vi "Text control 2 v5.0_pump-specific.vi"() -> ()   [LabVIEW 2016]
panel:
  in  "Tab Control":enum32{"Main", "Other parameters"}(tab)
  out "Line running":i32
  out "Total lines":i32
  out "Path":path=path "C:/users/rlp38/09Apr2009LTtesting/test2.txt"
  out "I vs Vg":cluster{"Y data in":dbl[], "X data in":dbl[]}[](graph)
  out "Is":dbl format="%.2e"
  out "Id":dbl format="%.2e"
  out "Ig":dbl format="%.2e"
  out "Id max vs time":cluster{"Y data in":dbl[], "X data in":dbl[]}[](graph)
  out "Id min vs time":cluster{"Y data in":dbl[], "X data in":dbl[]}[](graph)
  out "I vs Vd":cluster{"Y data in":dbl[], "X data in":dbl[]}[](graph)
  in  "Program":string="#-------------------------------------------------------\n# Liquid cycling script\n# Version 0.1\n# Author: Dimitrios Simatos\n# Last updated: 2017-10-12\n#-------------------------------------------------------\n# Things to do before running the script:\n# Set time units to minutes.\n# Set filenames.\n# Replace the tubing, if necessary.\n#-------------------------------------------------------\n# Port connections\n# Port 1: Waste\n# Port 2: Device\n# Port 3: Ultrapure water\n# Port 4: Nothing\n# Port 5: Nothing\n# Port 6: Nothing\n#-------------------------------------------------------\n# Execution time: 4 x 30 = 120 minutes = 2 hours\n# This script is designed to perform a cycling experiment between two liquids.\n# There are 4 pumping cycles, each one followed by 30 minutes of measurements.\n# All cycles pump ultrapure water (port 3).\n# Flow V = 20 pulses/second (400 ul/min)\n#-------------------------------------------------------\n# Cycle 1\npump /1ZR #initialize pump\npump /1Q #query pump\ntransfer d 1 -1 -0.1 -1 -1 0\npump /1? #report absolute plunger position\npump /1?6 #report valve position\nwait-min 1 #wait 1 minute\ntransfer d 1 -1 -0.1 -1 -1 0\npump /1N0R #set step resolution: 0.01 mm\npump /1Q #query pump\npump /1? #report absolute plunger position (the plunger should be at 0)\npump /1?6 #report valve position\nwait 1000 #wait 1 second\npump /1V300R #choose speed: 300 steps/s\npump /1Q #query pump\nwait 1000 #wait 1 second\npump /1O3R #go to port 3, counterclockwise rotation\npump /1Q #query pump\nwait 1000 #wait 1 second\npump /1A2400R #go to absolute position 2400\nwait 20000 #wait 20 seconds\npump /1V20R #set speed to 20 steps/s\npump /1Q #query pump\nwait 10000 # wait 10 seconds\ntransfer d 1 -1 -0.1 -1 -1 0\npump /1? #report absolute plunger position (the plunger should have finished moving)\npump /1?6 #report valve position\npump /1O2R #switch to port 2, counterclockwise rotation\npump /1Q #query pump\nwait 200 #wait 200 milliseconds\npump /1A0R #go to absolute position 0 (= empty syringe)\npump /1Q #query pump\npump /1? #report absolute plunger position (the plunger should be moving to 0)\npump /1?6 #report valve position\ntransfer d 1 -1 -0.1 -1 -1 0\nwait-min 1\npump /1Q #query pump\npump /1? #report absolute plunger position (the plunger should be moving to 0)\npump /1?6 #report valve position\ntransfer d 1 -1 -0.1 -1 -1 0\nwait-min 1\npump /1Q #query pump\npump /1? #report absolute plunger position\npump /1?6 #report valve position\ntransfer d 1 -1 -0.1 -1 -1 0\nwait-min 1\npump /1Q #query pump\npump /1? #report absolute plunger position\npump /1?6 #report valve position\ntransfer d 1 -1 -0.1 -1 -1 0\nwait-min 1\npump /1Q #query pump\npump /1? #report absolute plunger position\npump /1?6 #report valve position\ntransfer d 1 -1 -0.1 -1 -1 0\nwait-min 1\npump /1Q #query pump\npump /1? #report absolute plunger position\npump /1?6 #report valve position\ntransfer d 1 -1 -0.1 -1 -1 0\nwait-min 1\npump /1Q #query pump\npump /1? #report absolute plunger position\npump /1?6 #report valve position\ntransfer d 1 -1 -0.1 -1 -1 0\nwait-min 1\npump /1Q #query pump\npump /1? #report absolute plunger position\npump /1?6 #report valve position\ntransfer d 1 -1 -0.1 -1 -1 0\nwait-min 1\npump /1Q #query pump\npump /1? #report absolute plunger position\npump /1?6 #report valve position\ntransfer d 1 -1 -0.1 -1 -1 0\nwait-min 1\npump /1Q #query pump\npump /1? #report absolute plunger position\npump /1?6 #report valve position\ntransfer d 1 -1 -0.1 -1 -1 0\nwait-min 1\npump /1Q #query pump\npump /1? #report absolute plunger position\npump /1?6 #report valve position\ntransfer d 1 -1 -0.1 -1 -1 0\nwait-min 1\npump /1Q #query pump\npump /1? #report absolute plunger position\npump /1?6 #report valve position\ntransfer d 1 -1 -0.1 -1 -1 0\nwait-min 1\npump /1Q #query pump\npump /1? #report absolute plunger position\npump /1?6 #report valve position\ntransfer d 1 -1 -0.1 -1 -1 0\nwait-min 1\npump /1Q #query pump\npump /1? #report absolute plunger position\npump /1?6 #report valve position\ntransfer d 1 -1 -0.1 -1 -1 0\nwait-min 1\npump /1Q #query pump\npump /1? #report absolute plunger position\npump /1?6 #report valve position\ntransfer d 1 -1 -0.1 -1 -1 0\nwait-min 1\npump /1Q #query pump\npump /1? #report absolute plunger position\npump /1?6 #report valve position\ntransfer d 1 -1 -0.1 -1 -1 0\nwait-min 1\npump /1Q #query pump\npump /1? #report absolute plunger position\npump /1?6 #report valve position\ntransfer d 1 -1 -0.1 -1 -1 0\nwait-min 1\npump /1Q #query pump\npump /1? #report absolute plunger position\npump /1?6 #report valve position\ntransfer d 1 -1 -0.1 -1 -1 0\nwait-min 1\npump /1Q #query pump\npump /1? #report absolute plunger position\npump /1?6 #report valve position\ntransfer d 1 -1 -0.1 -1 -1 0\nwait-min 1\npump /1Q #query pump\npump /1? #report absolute plunger position\npump /1?6 #report valve position\ntransfer d 1 -1 -0.1 -1 -1 0\nwait-min 1\npump /1Q #query pump\npump /1? #report absolute plunger position\npump /1?6 #report valve position\ntransfer d 1 -1 -0.1 -1 -1 0\nwait-min 1\npump /1Q #query pump\npump /1? #report absolute plunger position\npump /1?6 #report valve position\ntransfer d 1 -1 -0.1 -1 -1 0\nwait-min 1\npump /1Q #query pump\npump /1? #report absolute plunger position\npump /1?6 #report valve position\ntransfer d 1 -1 -0.1 -1 -1 0\nwait-min 1\npump /1Q #query pump\npump /1? #report absolute plunger position\npump /1?6 #report valve position\ntransfer d 1 -1 -0.1 -1 -1 0\nwait-min 1\npump /1Q #query pump\npump /1? #report absolute plunger position\npump /1?6 #report valve position\ntransfer d 1 -1 -0.1 -1 -1 0\nwait-min 1\n#-------------------------------------------------------\n# Cycle 2\npump /1ZR #initialize pump\npump /1Q #query pump\ntransfer d 1 -1 -0.1 -1 -1 0\npump /1? #report absolute plunger position\npump /1?6 #report valve position\nwait-min 1 #wait 1 minute\ntransfer d 1 -1 -0.1 -1 -1 0\npump /1N0R #set step resolution: 0.01 mm\npump /1Q #query pump\npump /1? #report absolute plunger position (the plunger should be at 0)\npump /1?6 #report valve position\nwait 1000 #wait 1 second\npump /1V300R #choose speed: 300 steps/s\npump /1Q #query pump\nwait 1000 #wait 1 second\npump /1O3R #go to port 3, counterclockwise rotation\npump /1Q #query pump\nwait 1000 #wait 1 second\npump /1A2400R #go to absolute position 2400\nwait 20000 #wait 20 seconds\ntransfer d 1 -1 -0.1 -1 -1 0\npump /1V20R #set speed to 20 steps/s\npump /1Q #query pump\nwait 10000 # wait 10 seconds\npump /1? #report absolute plunger position (the plunger should have finished moving)\npump /1?6 #report valve position\npump /1O2R #switch to port 2, counterclockwise rotation\npump /1Q #query pump\nwait 200 #wait 200 milliseconds\npump /1A0R #go to absolute position 0 (= empty syringe)\npump /1Q #query pump\npump /1? #report absolute plunger position (the plunger should be moving to 0)\npump /1?6 #report valve position\ntransfer d 1 -1 -0.1 -1 -1 0\nwait-min 1\npump /1Q #query pump\npump /1? #report absolute plunger position (the plunger should be moving to 0)\npump /1?6 #report valve position\ntransfer d 1 -1 -0.1 -1 -1 0\nwait-min 1\npump /1Q #query pump\npump /1? #report absolute plunger position\npump /1?6 #report valve position\ntransfer d 1 -1 -0.1 -1 -1 0\nwait-min 1\npump /1Q #query pump\npump /1? #report absolute plunger position\npump /1?6 #report valve position\ntransfer d 1 -1 -0.1 -1 -1 0\nwait-min 1\npump /1Q #query pump\npump /1? #report absolute plunger position\npump /1?6 #report valve position\ntransfer d 1 -1 -0.1 -1 -1 0\nwait-min 1\npump /1Q #query pump\npump /1? #report absolute plunger position\npump /1?6 #report valve position\ntransfer d 1 -1 -0.1 -1 -1 0\nwait-min 1\npump /1Q #query pump\npump /1? #report absolute plunger position\npump /1?6 #report valve position\ntransfer d 1 -1 -0.1 -1 -1 0\nwait-min 1\npump /1Q #query pump\npump /1? #report absolute plunger position\npump /1?6 #report valve position\ntransfer d 1 -1 -0.1 -1 -1 0\nwait-min 1\npump /1Q #query pump\npump /1? #report absolute plunger position\npump /1?6 #report valve position\ntransfer d 1 -1 -0.1 -1 -1 0\nwait-min 1\npump /1Q #query pump\npump /1? #report absolute plunger position\npump /1?6 #report valve position\ntransfer d 1 -1 -0.1 -1 -1 0\nwait-min 1\npump /1Q #query pump\npump /1? #report absolute plunger position\npump /1?6 #report valve position\ntransfer d 1 -1 -0.1 -1 -1 0\nwait-min 1\npump /1Q #query pump\npump /1? #report absolute plunger position\npump /1?6 #report valve position\ntransfer d 1 -1 -0.1 -1 -1 0\nwait-min 1\npump /1Q #query pump\npump /1? #report absolute plunger position\npump /1?6 #report valve position\ntransfer d 1 -1 -0.1 -1 -1 0\nwait-min 1\npump /1Q #query pump\npump /1? #report absolute plunger position\npump /1?6 #report valve position\ntransfer d 1 -1 -0.1 -1 -1 0\nwait-min 1\npump /1Q #query pump\npump /1? #report absolute plunger position\npump /1?6 #report valve position\ntransfer d 1 -1 -0.1 -1 -1 0\nwait-min 1\npump /1Q #query pump\npump /1? #report absolute plunger position\npump /1?6 #report valve position\ntransfer d 1 -1 -0.1 -1 -1 0\nwait-min 1\npump /1Q #query pump\npump /1? #report absolute plunger position\npump /1?6 #report valve position\ntransfer d 1 -1 -0.1 -1 -1 0\nwait-min 1\npump /1Q #query pump\npump /1? #report absolute plunger position\npump /1?6 #report valve position\ntransfer d 1 -1 -0.1 -1 -1 0\nwait-min 1\npump /1Q #query pump\npump /1? #report absolute plunger position\npump /1?6 #report valve position\ntransfer d 1 -1 -0.1 -1 -1 0\nwait-min 1\npump /1Q #query pump\npump /1? #report absolute plunger position\npump /1?6 #report valve position\ntransfer d 1 -1 -0.1 -1 -1 0\nwait-min 1\npump /1Q #query pump\npump /1? #report absolute plunger position\npump /1?6 #report valve position\ntransfer d 1 -1 -0.1 -1 -1 0\nwait-min 1\npump /1Q #query pump\npump /1? #report absolute plunger position\npump /1?6 #report valve position\ntransfer d 1 -1 -0.1 -1 -1 0\nwait-min 1\npump /1Q #query pump\npump /1? #report absolute plunger position\npump /1?6 #report valve position\ntransfer d 1 -1 -0.1 -1 -1 0\nwait-min 1\npump /1Q #query pump\npump /1? #report absolute plunger position\npump /1?6 #report valve position\ntransfer d 1 -1 -0.1 -1 -1 0\nwait-min 1\npump /1Q #query pump\npump /1? #report absolute plunger position\npump /1?6 #report valve position\ntransfer d 1 -1 -0.1 -1 -1 0\nwait-min 1\n#-------------------------------------------------------\n# Cycle 3\npump /1ZR #initialize pump\npump /1Q #query pump\ntransfer d 1 -1 -0.1 -1 -1 0\npump /1? #report absolute plunger position\npump /1?6 #report valve position\nwait-min 1 #wait 1 minute\ntransfer d 1 -1 -0.1 -1 -1 0\npump /1N0R #set step resolution: 0.01 mm\npump /1Q #query pump\npump /1? #report absolute plunger position (the plunger should be at 0)\npump /1?6 #report valve position\nwait 1000 #wait 1 second\npump /1V300R #choose speed: 300 steps/s\npump /1Q #query pump\nwait 1000 #wait 1 second\npump /1O3R #go to port 3, counterclockwise rotation\npump /1Q #query pump\nwait 1000 #wait 1 second\npump /1A2400R #go to absolute position 2400\nwait 20000 #wait 20 seconds\ntransfer d 1 -1 -0.1 -1 -1 0\npump /1V20R #set speed to 20 steps/s\npump /1Q #query pump\nwait 10000 # wait 10 seconds\npump /1? #report absolute plunger position (the plunger should have finished moving)\npump /1?6 #report valve position\npump /1O2R #switch to port 2, counterclockwise rotation\npump /1Q #query pump\nwait 200 #wait 200 milliseconds\npump /1A0R #go to absolute position 0 (= empty syringe)\npump /1Q #query pump\npump /1? #report absolute plunger position (the plunger should be moving to 0)\npump /1?6 #report valve position\ntransfer d 1 -1 -0.1 -1 -1 0\nwait-min 1\npump /1Q #query pump\npump /1? #report absolute plunger position (the plunger should be moving to 0)\npump /1?6 #report valve position\ntransfer d 1 -1 -0.1 -1 -1 0\nwait-min 1\npump /1Q #query pump\npump /1? #report absolute plunger position\npump /1?6 #report valve position\ntransfer d 1 -1 -0.1 -1 -1 0\nwait-min 1\npump /1Q #query pump\npump /1? #report absolute plunger position\npump /1?6 #report valve position\ntransfer d 1 -1 -0.1 -1 -1 0\nwait-min 1\npump /1Q #query pump\npump /1? #report absolute plunger position\npump /1?6 #report valve position\ntransfer d 1 -1 -0.1 -1 -1 0\nwait-min 1\npump /1Q #query pump\npump /1? #report absolute plunger position\npump /1?6 #report valve position\ntransfer d 1 -1 -0.1 -1 -1 0\nwait-min 1\npump /1Q #query pump\npump /1? #report absolute plunger position\npump /1?6 #report valve position\ntransfer d 1 -1 -0.1 -1 -1 0\nwait-min 1\npump /1Q #query pump\npump /1? #report absolute plunger position\npump /1?6 #report valve position\ntransfer d 1 -1 -0.1 -1 -1 0\nwait-min 1\npump /1Q #query pump\npump /1? #report absolute plunger position\npump /1?6 #report valve position\ntransfer d 1 -1 -0.1 -1 -1 0\nwait-min 1\npump /1Q #query pump\npump /1? #report absolute plunger position\npump /1?6 #report valve position\ntransfer d 1 -1 -0.1 -1 -1 0\nwait-min 1\npump /1Q #query pump\npump /1? #report absolute plunger position\npump /1?6 #report valve position\ntransfer d 1 -1 -0.1 -1 -1 0\nwait-min 1\npump /1Q #query pump\npump /1? #report absolute plunger position\npump /1?6 #report valve position\ntransfer d 1 -1 -0.1 -1 -1 0\nwait-min 1\npump /1Q #query pump\npump /1? #report absolute plunger position\npump /1?6 #report valve position\ntransfer d 1 -1 -0.1 -1 -1 0\nwait-min 1\npump /1Q #query pump\npump /1? #report absolute plunger position\npump /1?6 #report valve position\ntransfer d 1 -1 -0.1 -1 -1 0\nwait-min 1\npump /1Q #query pump\npump /1? #report absolute plunger position\npump /1?6 #report valve position\ntransfer d 1 -1 -0.1 -1 -1 0\nwait-min 1\npump /1Q #query pump\npump /1? #report absolute plunger position\npump /1?6 #report valve position\ntransfer d 1 -1 -0.1 -1 -1 0\nwait-min 1\npump /1Q #query pump\npump /1? #report absolute plunger position\npump /1?6 #report valve position\ntransfer d 1 -1 -0.1 -1 -1 0\nwait-min 1\npump /1Q #query pump\npump /1? #report absolute plunger position\npump /1?6 #report valve position\ntransfer d 1 -1 -0.1 -1 -1 0\nwait-min 1\npump /1Q #query pump\npump /1? #report absolute plunger position\npump /1?6 #report valve position\ntransfer d 1 -1 -0.1 -1 -1 0\nwait-min 1\npump /1Q #query pump\npump /1? #report absolute plunger position\npump /1?6 #report valve position\ntransfer d 1 -1 -0.1 -1 -1 0\nwait-min 1\npump /1Q #query pump\npump /1? #report absolute plunger position\npump /1?6 #report valve position\ntransfer d 1 -1 -0.1 -1 -1 0\nwait-min 1\npump /1Q #query pump\npump /1? #report absolute plunger position\npump /1?6 #report valve position\ntransfer d 1 -1 -0.1 -1 -1 0\nwait-min 1\npump /1Q #query pump\npump /1? #report absolute plunger position\npump /1?6 #report valve position\ntransfer d 1 -1 -0.1 -1 -1 0\nwait-min 1\npump /1Q #query pump\npump /1? #report absolute plunger position\npump /1?6 #report valve position\ntransfer d 1 -1 -0.1 -1 -1 0\nwait-min 1\npump /1Q #query pump\npump /1? #report absolute plunger position\npump /1?6 #report valve position\ntransfer d 1 -1 -0.1 -1 -1 0\nwait-min 1\n#-------------------------------------------------------\n# Cycle 4\npump /1ZR #initialize pump\npump /1Q #query pump\ntransfer d 1 -1 -0.1 -1 -1 0\npump /1? #report absolute plunger position\npump /1?6 #report valve position\nwait-min 1 #wait 1 minute\ntransfer d 1 -1 -0.1 -1 -1 0\npump /1N0R #set step resolution: 0.01 mm\npump /1Q #query pump\npump /1? #report absolute plunger position (the plunger should be at 0)\npump /1?6 #report valve position\nwait 1000 #wait 1 second\npump /1V300R #choose speed: 300 steps/s\npump /1Q #query pump\nwait 1000 #wait 1 second\npump /1O3R #go to port 3, counterclockwise rotation\npump /1Q #query pump\nwait 1000 #wait 1 second\npump /1A2400R #go to absolute position 2400\nwait 20000 #wait 20 seconds\ntransfer d 1 -1 -0.1 -1 -1 0\npump /1V20R #set speed to 20 steps/s\npump /1Q #query pump\nwait 10000 # wait 10 seconds\npump /1? #report absolute plunger position (the plunger should have finished moving)\npump /1?6 #report valve position\npump /1O2R #switch to port 2, counterclockwise rotation\npump /1Q #query pump\nwait 200 #wait 200 milliseconds\npump /1A0R #go to absolute position 0 (= empty syringe)\npump /1Q #query pump\npump /1? #report absolute plunger position (the plunger should be moving to 0)\npump /1?6 #report valve position\ntransfer d 1 -1 -0.1 -1 -1 0\nwait-min 1\npump /1Q #query pump\npump /1? #report absolute plunger position (the plunger should be moving to 0)\npump /1?6 #report valve position\ntransfer d 1 -1 -0.1 -1 -1 0\nwait-min 1\npump /1Q #query pump\npump /1? #report absolute plunger position\npump /1?6 #report valve position\ntransfer d 1 -1 -0.1 -1 -1 0\nwait-min 1\npump /1Q #query pump\npump /1? #report absolute plunger position\npump /1?6 #report valve position\ntransfer d 1 -1 -0.1 -1 -1 0\nwait-min 1\npump /1Q #query pump\npump /1? #report absolute plunger position\npump /1?6 #report valve position\ntransfer d 1 -1 -0.1 -1 -1 0\nwait-min 1\npump /1Q #query pump\npump /1? #report absolute plunger position\npump /1?6 #report valve position\ntransfer d 1 -1 -0.1 -1 -1 0\nwait-min 1\npump /1Q #query pump\npump /1? #report absolute plunger position\npump /1?6 #report valve position\ntransfer d 1 -1 -0.1 -1 -1 0\nwait-min 1\npump /1Q #query pump\npump /1? #report absolute plunger position\npump /1?6 #report valve position\ntransfer d 1 -1 -0.1 -1 -1 0\nwait-min 1\npump /1Q #query pump\npump /1? #report absolute plunger position\npump /1?6 #report valve position\ntransfer d 1 -1 -0.1 -1 -1 0\nwait-min 1\npump /1Q #query pump\npump /1? #report absolute plunger position\npump /1?6 #report valve position\ntransfer d 1 -1 -0.1 -1 -1 0\nwait-min 1\npump /1Q #query pump\npump /1? #report absolute plunger position\npump /1?6 #report valve position\ntransfer d 1 -1 -0.1 -1 -1 0\nwait-min 1\npump /1Q #query pump\npump /1? #report absolute plunger position\npump /1?6 #report valve position\ntransfer d 1 -1 -0.1 -1 -1 0\nwait-min 1\npump /1Q #query pump\npump /1? #report absolute plunger position\npump /1?6 #report valve position\ntransfer d 1 -1 -0.1 -1 -1 0\nwait-min 1\npump /1Q #query pump\npump /1? #report absolute plunger position\npump /1?6 #report valve position\ntransfer d 1 -1 -0.1 -1 -1 0\nwait-min 1\npump /1Q #query pump\npump /1? #report absolute plunger position\npump /1?6 #report valve position\ntransfer d 1 -1 -0.1 -1 -1 0\nwait-min 1\npump /1Q #query pump\npump /1? #report absolute plunger position\npump /1?6 #report valve position\ntransfer d 1 -1 -0.1 -1 -1 0\nwait-min 1\npump /1Q #query pump\npump /1? #report absolute plunger position\npump /1?6 #report valve position\ntransfer d 1 -1 -0.1 -1 -1 0\nwait-min 1\npump /1Q #query pump\npump /1? #report absolute plunger position\npump /1?6 #report valve position\ntransfer d 1 -1 -0.1 -1 -1 0\nwait-min 1\npump /1Q #query pump\npump /1? #report absolute plunger position\npump /1?6 #report valve position\ntransfer d 1 -1 -0.1 -1 -1 0\nwait-min 1\npump /1Q #query pump\npump /1? #report absolute plunger position\npump /1?6 #report valve position\ntransfer d 1 -1 -0.1 -1 -1 0\nwait-min 1\npump /1Q #query pump\npump /1? #report absolute plunger position\npump /1?6 #report valve position\ntransfer d 1 -1 -0.1 -1 -1 0\nwait-min 1\npump /1Q #query pump\npump /1? #report absolute plunger position\npump /1?6 #report valve position\ntransfer d 1 -1 -0.1 -1 -1 0\nwait-min 1\npump /1Q #query pump\npump /1? #report absolute plunger position\npump /1?6 #report valve position\ntransfer d 1 -1 -0.1 -1 -1 0\nwait-min 1\npump /1Q #query pump\npump /1? #report absolute plunger position\npump /1?6 #report valve position\ntransfer d 1 -1 -0.1 -1 -1 0\nwait-min 1\npump /1Q #query pump\npump /1? #report absolute plunger position\npump /1?6 #report valve position\ntransfer d 1 -1 -0.1 -1 -1 0\nwait-min 1\n#-------------------------------------------------------"
  out "Command running:":string="#output s 0 0 0 -0.008 0.008 0.002"
  out "Serial port data":string
  out "Elapsed Time":dbl caption="Elapsed Time (s)"
  in  "Units":u16(ring)=1 items=["Seconds", "Minutes", "Hours"]
  in  "Time Offset":dbl caption="Set Start Time (s)"
  in  "Reset":bool
  in  "Auto Reset":bool
  in  "integration time":u32(slide) max=2 step=1 scale=0.0..2.0
  in  "Interrupt run":bool
  out "Absolute plunger position vs time":cluster{"Y data in":dbl[], "X data in":dbl[]}[](graph)
  out "Valve position vs time":cluster{"Y data in":dbl[], "X data in":dbl[]}[](graph)
  in  "Halt pump":bool
  in  "Hard stop pump":bool
  in  "Gate Range\nmode":u16(ring) items=["Auto", "Limited", "Fixed"]
  in  "Gate Range":u8(slide)=6 max=11 scale=0.0..11.0
  in  "Source/Drain\nRange mode":u16(ring) items=["Auto", "Limited", "Fixed"]
  in  "Source/Drain Range":u8(slide)=6 max=11 scale=0.0..11.0
  in  "Panel Controls":T1={"Emergency Stop"=refnum, "TransGraph Max"=1e-05, "Text/Graph (text=false)"=TRUE} {"TransGraph Max" format="%.2e"}
  in  "Panel Controls 2":T2={"Emergency Stop"=refnum, "TransGraph Max"=1e-05, "Text/Graph (text=false)"=TRUE, "TransGraph Min"=1e-11} {"TransGraph Min" format="%.2e"; "TransGraph Max" format="%.2e"}
  in  "SMU4":cluster{"on/off":bool, "Voltage":dbl} {"Voltage" min=-100.0 max=100.0 format="%.2f"}
  in  "Full Reset":bool
  in  "Standby":T3
  out "error out":errorcluster
  in  "Delay before read (ms)":u32=1000
  in  "byte count":u32=64
  in  "Serial End Mode for Reads":u16(ring)=2 items=["None", "LastBit", "TermChar"]
  in  "Timeout (ms)":u32=10000
  in  "Enable Termination\nChar (T)":bool=TRUE
  in  "Termination char\n(0xA = '\\n' = LF)\n(0xD = '\\r' = CR)":u8=13 format="%.0x"
  in  "flow control":u16(ring) items=["None"=0, "XON/XOFF"=1, "RTS/CTS"=2, "DTR/DSR"=4]
  in  "stop bits":u16(ring)=10 items=["1.0"=10, "1.5"=15, "2.0"=20]
  in  "parity":u16(ring) items=["None", "Odd", "Even", "Mark", "Space"]
  in  "data bits":u16=8 min=5 max=8 step=1
  in  "VISA resource name":refnum<visa-resource-name>="COM6"
  in  "baud rate":u32=9600
  in  "Drain: Compliance":dbl=0.001 format="%.8f"
  in  "Gate: Compliance":dbl=0.001 format="%.8f"
  in  "hold time /s":dbl format="%.2f"
  in  "delay time /s":dbl format="%.2f"
  in  "Integration time (short)":dbl=0.0019 min=8e-05 max=0.0019 step=8e-05 format="%^.0e"
  in  "Integration time (long)":dbl=0.32 min=0.04 max=2.0 step=0.02 format="%.2f"
  in  "Step delay /s":dbl format="%.2f"
  in  "Prefix (transfer)":string="_step_1_ultrapure_H2O_"
  in  "Suffix (transfer)":string="_T.txt"
  in  "Prefix (Idmax-Idmin)":string="_step_1_ultrapure_H2O_Idmax_Idmin_vs_time_Vg=-1.0V_Vd=-1.0V"
  in  "Suffix (Idmax-Idmin)":string=".txt"
  in  "Prefix (output)":string="_step_1_ultrapure_H2O_"
  in  "Suffix (output)":string="_O.txt"
  in  "Prefix (script)":string="_step_1_ultrapure_H2O_script"
  in  "Prefix (serial port log)":string="_step_1_ultrapure_H2O_serial port output"
  in  "Prefix (plunger)":string="_step_1_ultrapure_H2O_plunger_vs_time"
  in  "Suffix (plunger)":string=".txt"
  in  "Prefix (valve)":string="_step_1_ultrapure_H2O_valve_vs_time"
  in  "Suffix (valve)":string=".txt"
  in  "Gate":T4={"Gate Start"=0.0, "Gate Stop"=2.0, "Gate Step (linear only)"=1.0, "Gate Compliance"=0.0001, "Gate PComp"=0.0, "Range mode"=0, "Range"=6} {"Range" max=11 scale=0.0..11.0; "Range mode" items=["Auto", "Limited", "Fixed"]; "Gate PComp" format="%^.2e"; "Gate Compliance" format="%^.2e"; "Gate Step (linear only)" format="%^.4e"; "Gate Stop" format="%^.4e"; "Gate Start" format="%^.4e"}
  in  "Drain 2":T5={"Drain Start"=0.0, "Drain Stop"=2.0, "Drain Compliance"=0.0001, "Drain Step"=1.0, "Drain PComp"=0.0, "Range mode"=0, "Range"=6} {"Range" max=11 scale=0.0..11.0; "Range mode" items=["Auto", "Limited", "Fixed"]; "Drain PComp" format="%^.2e"; "Drain Step" format="%^.4e"; "Drain Compliance" format="%^.2e"; "Drain Stop" format="%^.4e"; "Drain Start" format="%^.4e"}
  in  "Timings 2":T6={"integration time"=0, "Short/Long integration time"=0.00064, "hold time (sec)"=0.0, "delay time (sec)"=0.0, "Step Time (0 disables)"=0.0, "sweep method"=0, "Pulse period"=0.005, "Base voltage"=0.0, "Pulse width"=0.0005} {"Pulse width" min=0.0005 max=0.1 step=0.0001 format="%.4f"; "Base voltage" format="%^.4e"; "Pulse period" min=0.005 max=1.0 step=0.0001 format="%.4f"; "sweep method" items=["Continuous", "Pulsed"]; "Step Time (0 disables)" format="%.2f"; "delay time (sec)" format="%.4f"; "hold time (sec)" format="%.4f"; "Short/Long integration time" format="%^.0e"; "integration time" scale=0.0..2.0}
  # "Syntax:\nitime [s|m|l]\ngaterangemode [a|l|f]\ndrainrangemode [a|l|f]\npulsed [on|off] PulsePeriod(sec) PulseBaseVoltage PulseONWidth(sec)\nstandby [on l off]\nwait NumMilliseconds\nwait-min NumMinutes\n# texthere = comment\ntransfer [s|d] VgStart VgStop VgStep VdStart VdStop VdStep\noutput [s|d] VgStart VgStop VgStep VdStart VdStop VdStep\nsample Vg Vd NumSamples Time(s) SampleInterval(s)\nsamplei Idg NumSamples Time(s) SampleInterval(s) VDGcompliance\n100 samples is approximately 13 seconds with medium integration\n# if in doubt use SampleInterval(s) = 0.004\nstressV VG VD IGcompliance IDcompliance Duration(sec)\nstressI IDG VDGcompliance Duration(sec)\nvsu2pulse Bias Duration(s)\npulsedstressV [s|d] VEstop VgON VgOFF Period(s) PulseONwidth(s) Vd\nsample-fpp Vg Vd NumSamples Time\nresample-fpp Vg Vd\ntransfer-fpp [s|d] VgStart VgStop VgStep VdStart VdStop VdStep\noutput-fpp [s|d] VgStart VgStop VgStep VdStart VdStop VdStep\nserial SerialPortCommand\npump SerialPortCommand for the OEM pump\n\nSPM OEM Pump Syntax (<x>: pump number, use 1 if only one pump):\nif the command syntax contains [R], then append the letter R to the command\n/<x>Q: query (a query command should follow each command)\n/<x>Z[R] or /<x>Y[R]: initialize pump\n/<x>N<n>[R] (<n>=0,1): <0> (<1>) microstep 0.01 mm (0.00125 mm) resolution\n/<x>I<n> (<n>=0-6): turn to port number n (clockwise)\n/<x>O<n> (<n>=0-6): turn to port number n (counterclockwise)\n/<x>X: Re-execute last command string\n/<x>G<n>[R] (<n>=0-60000): repeat command sequence (default: 0, 0=loop forever)\n/<x>g: Mark the start of a repeat sequence (max = 10)\n/<x>M<n>[R] (<n>=0-86400000): delay command execution by n milliseconds\n/<x>H: Halt; Pause the sequence after finishing the current move\n/<x>T: Hardstop; Interrupt the current move and suppress it from the sequence\n/<x>A<n>[R] (<n>=0-3000 with N=0, 0-24000 with N=1): absolute position\n/<x>P<n>[R] (<n>=0-3000 with N=0, 0-24000 with N=1): relative pickup\n/<x>D<n>[R] (<n>=0-3000 with N=0, 0-24000 with N=1): relative dispense\n/<x>V<n>[R] (<n>=5-1600 default: 150): set peak speed (pulses/sec)\n/<x>S<n>[R] (<n>=10-40 default: 22): set speed (NOT in pulses/sec, look in manual)\nNOTE: When controlled with absolute position, one does not need to pay special attention to the syringe that is mounted on the pump.\nWithdraw from lower stage (ports 3, 5), dispense from higher stage (ports 2, 4, 6).\nConnect Port 1 to waste."
  # "Time"
  # "1\n2\n3\n4\n5\n6\n7\n8\n9\n10\n11\n12\n13\n14\n15\n16\n17\n18\n19\n20"
  # "Serial port settings"
  # "Filename settings"
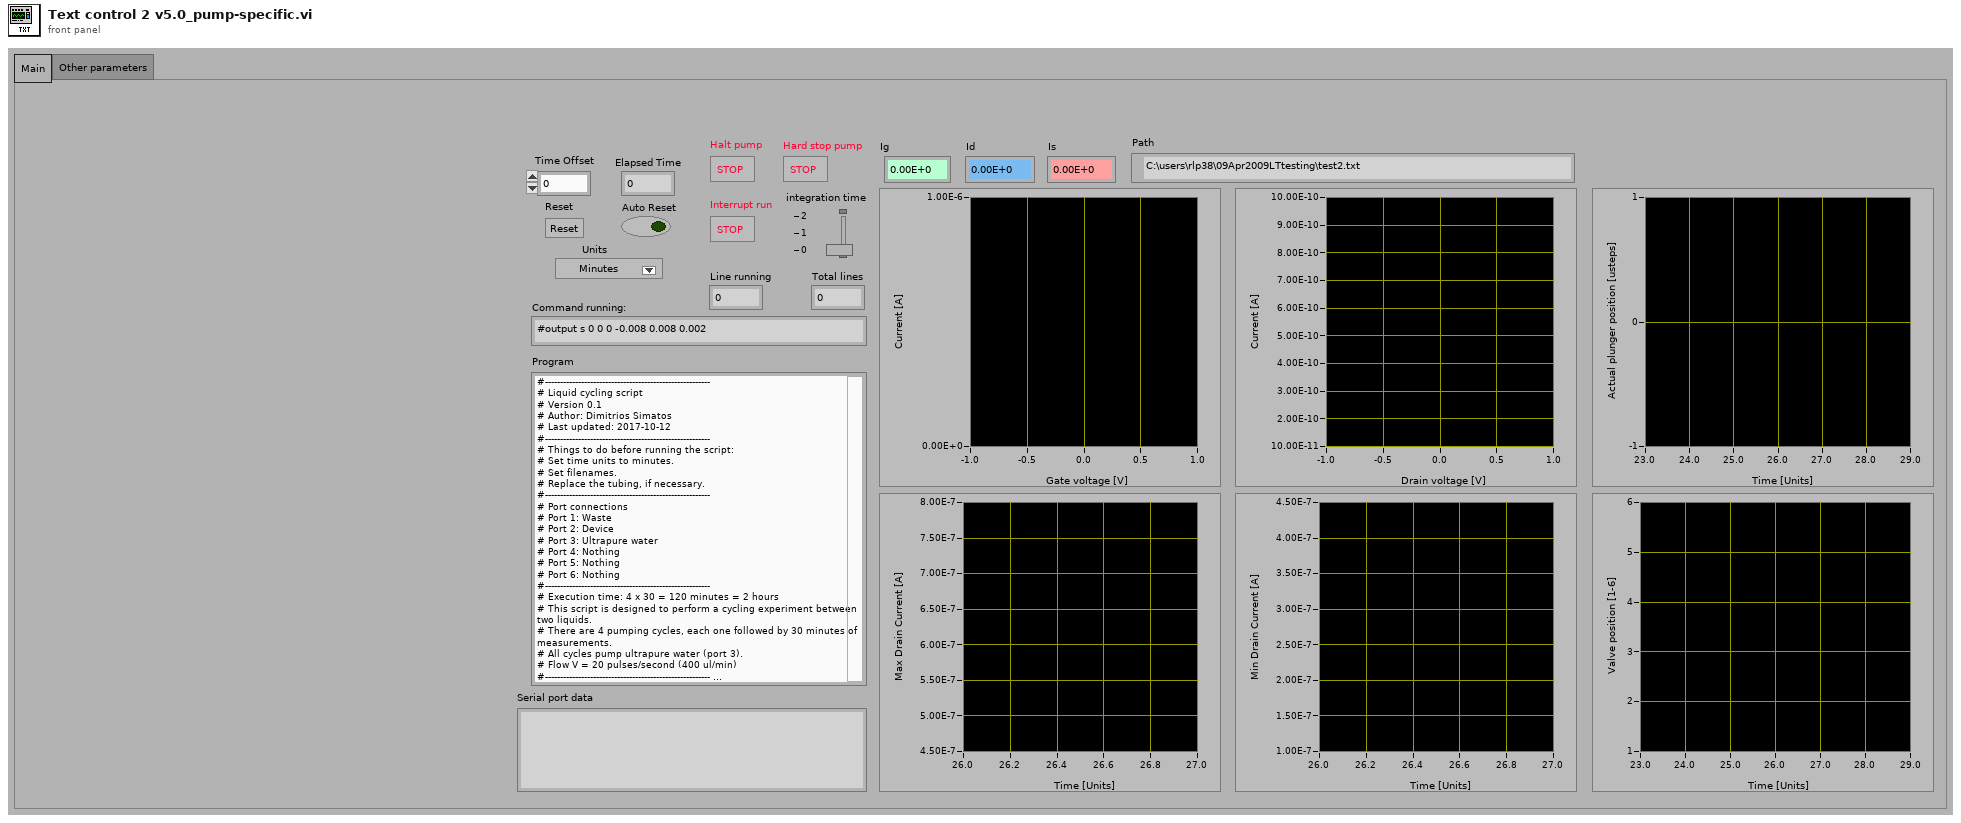
[diagram p1: front panel]
types:
  T1 = cluster{"Emergency Stop":refnum<vi>, "TransGraph Max":dbl, "Text/Graph (text=false)":bool}
  T2 = cluster{"Emergency Stop":refnum<vi>, "TransGraph Max":dbl, "Text/Graph (text=false)":bool, "TransGraph Min":dbl}
  T3 = cluster{"Gate Standby":bool, "Drain Standby":bool}
  T4 = cluster{"Gate Start":dbl, "Gate Stop":dbl, "Gate Step (linear only)":dbl, "Gate Compliance":dbl, "Gate PComp":dbl, "Range mode":u16, "Range":u8}
  T5 = cluster{"Drain Start":dbl, "Drain Stop":dbl, "Drain Compliance":dbl, "Drain Step":dbl, "Drain PComp":dbl, "Range mode":u16, "Range":u8}
  T6 = cluster{"integration time":u32, "Short/Long integration time":dbl, "hold time (sec)":dbl, "delay time (sec)":dbl, "Step Time (0 disables)":dbl, "sweep method":u16, "Pulse period":dbl, "Base voltage":dbl, "Pulse width":dbl}
  T7 = enum16{"open", "replace", "create", "open or create", "replace or create", "replace or create with confirmation"}
  T8 = cluster{"V2 Start":dbl, "V2 Step":dbl, "Number of points":i32}
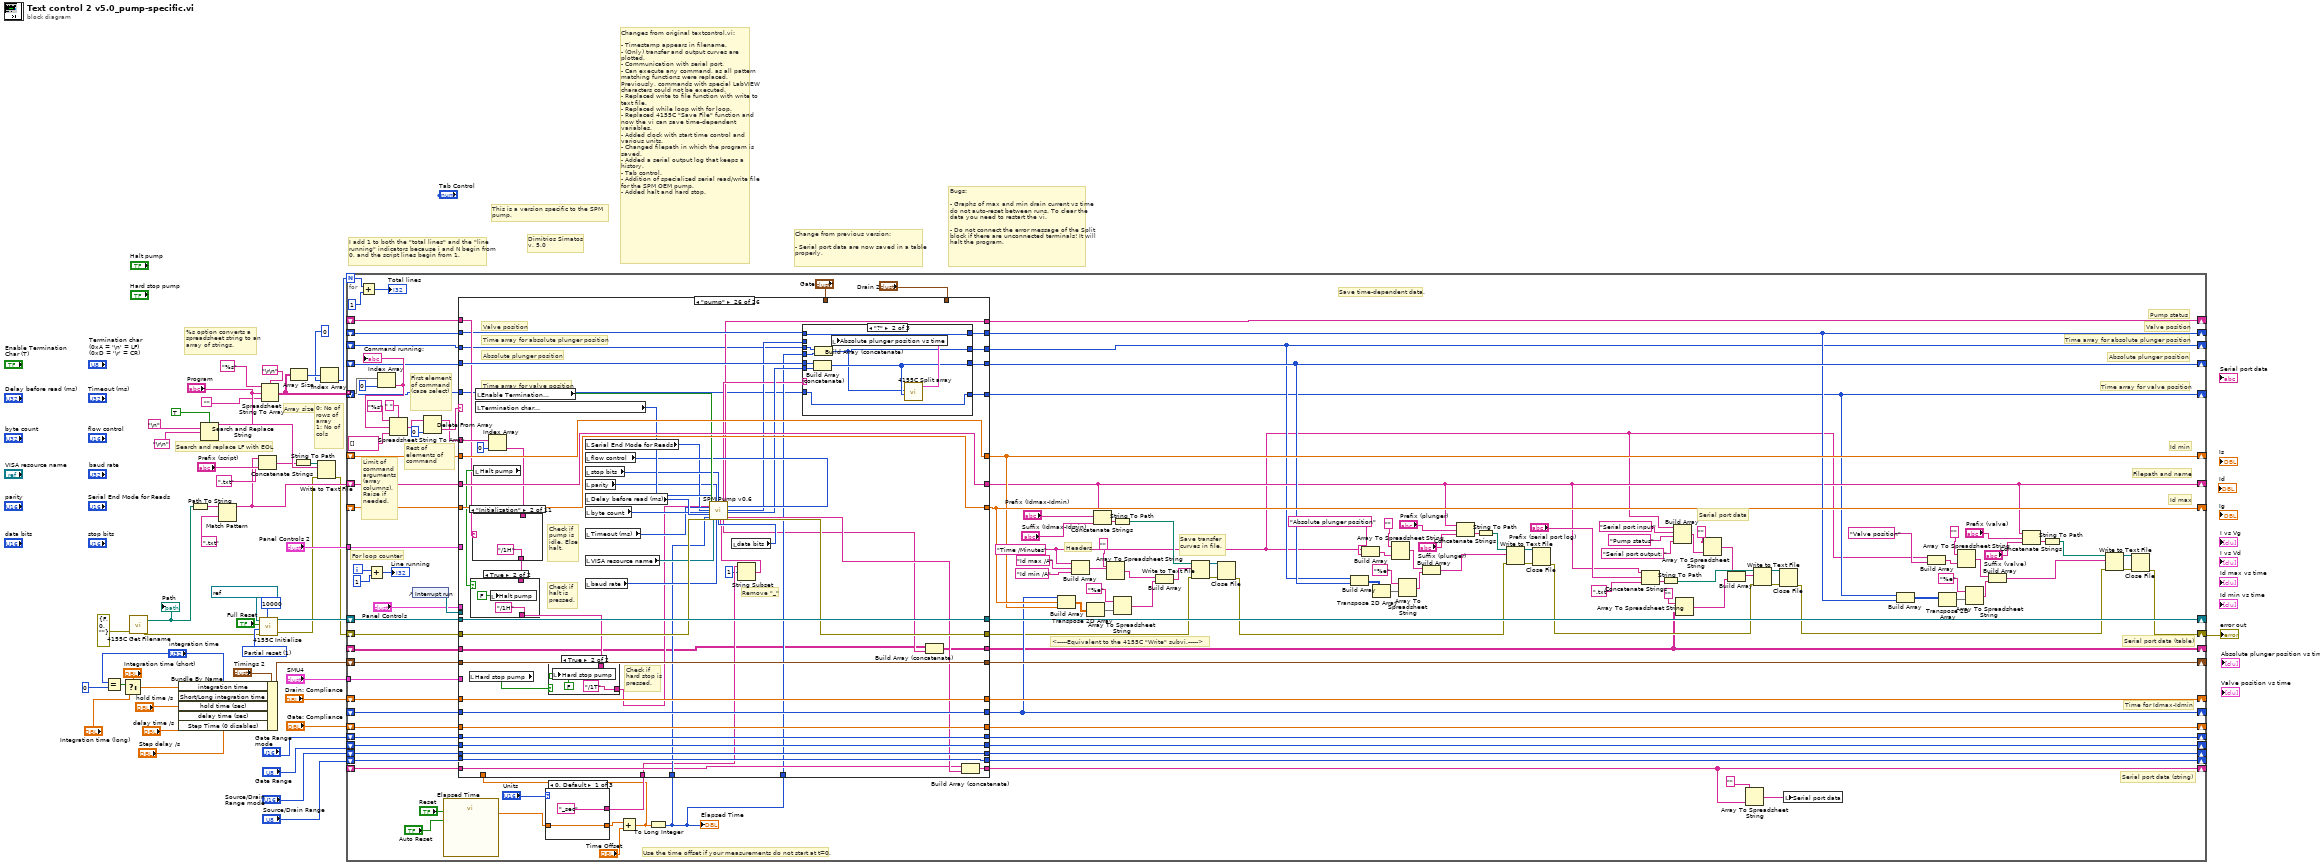
[diagram p0: block diagram]
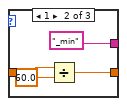
[diagram p2: hidden frame]
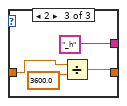
[diagram p3: hidden frame]
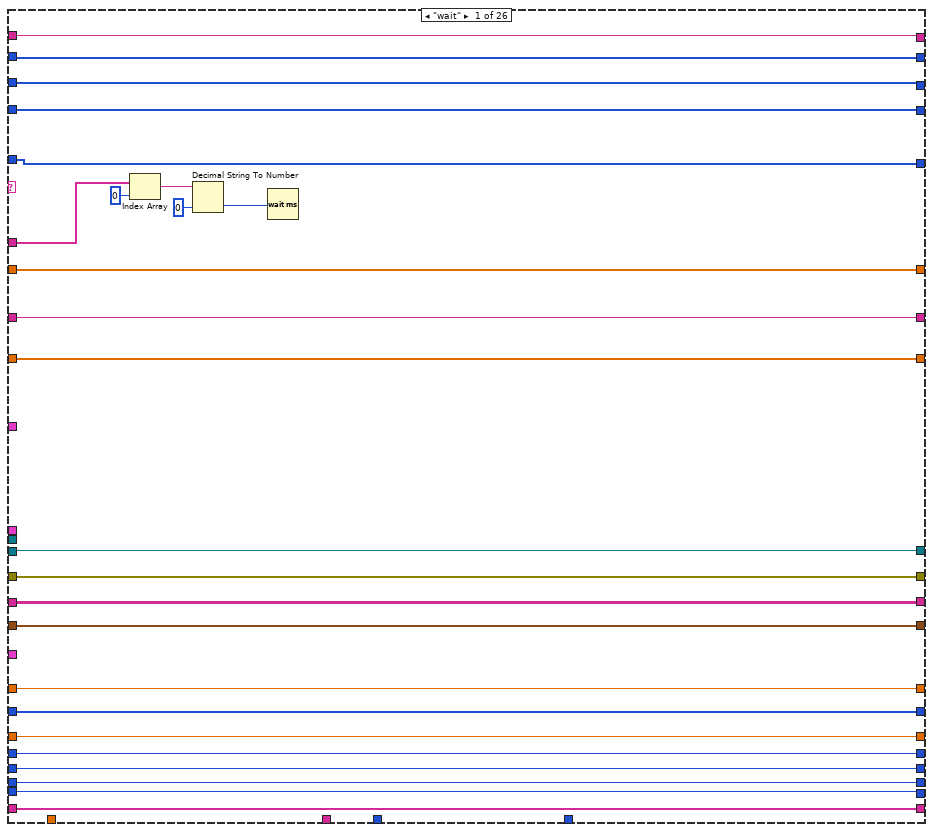
[diagram p4: hidden frame]
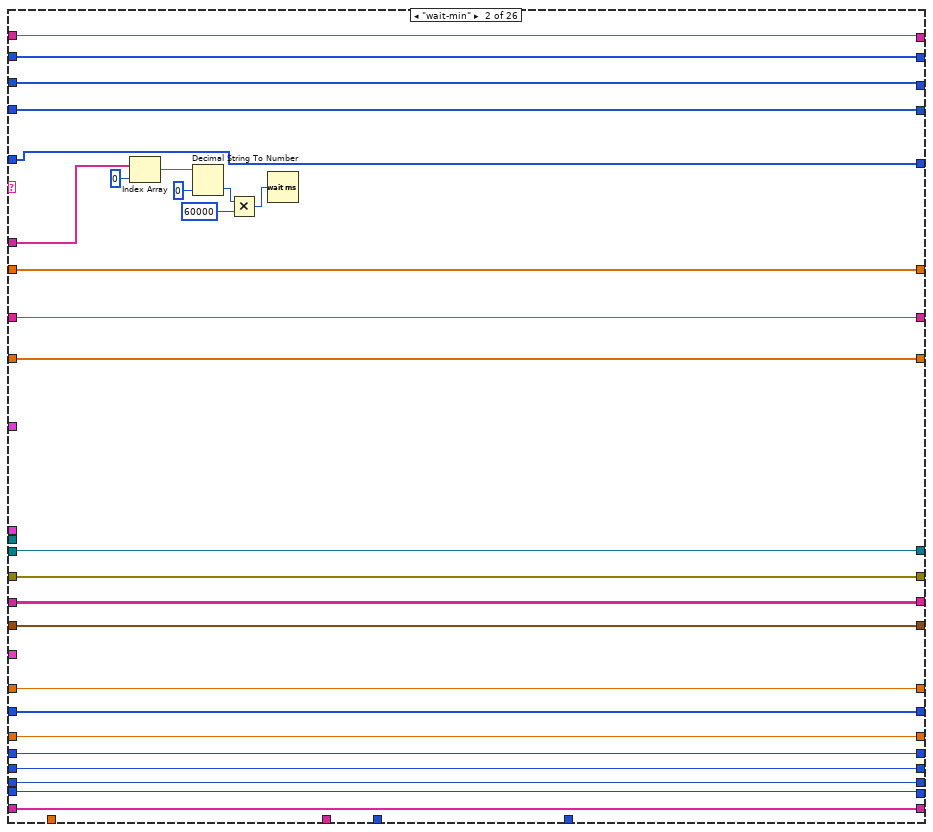
[diagram p5: hidden frame]
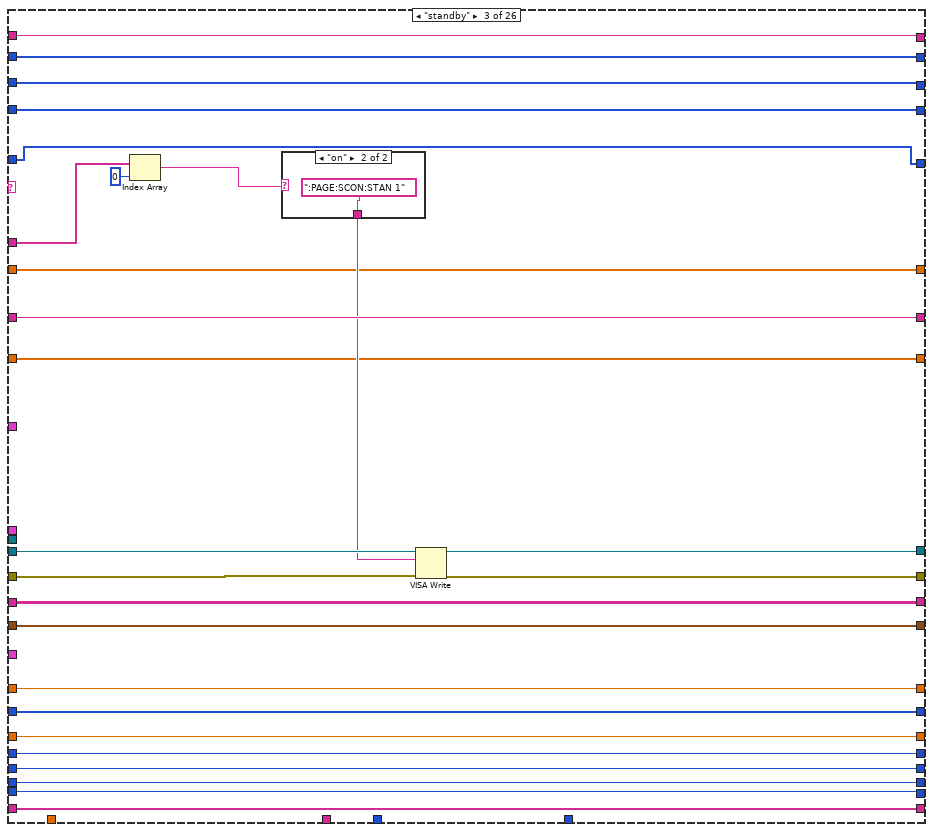
[diagram p6: hidden frame]
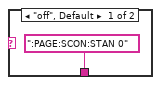
[diagram p7: hidden frame]
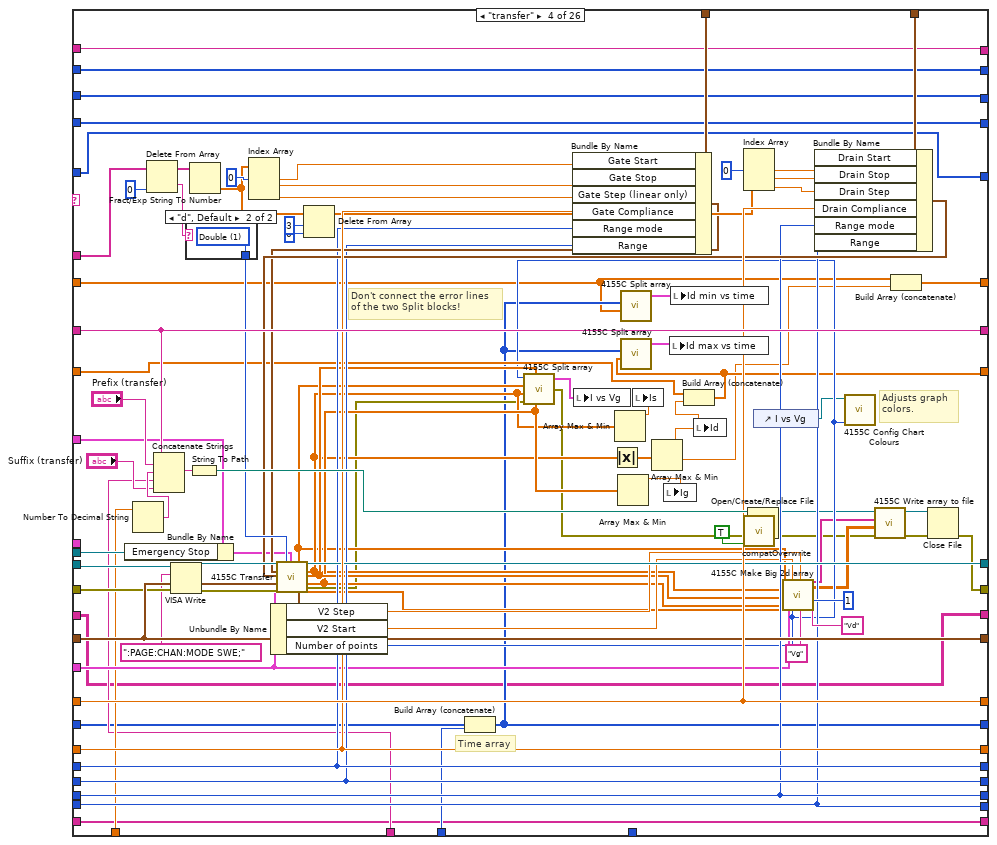
[diagram p8: hidden frame]
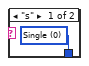
[diagram p9: hidden frame]
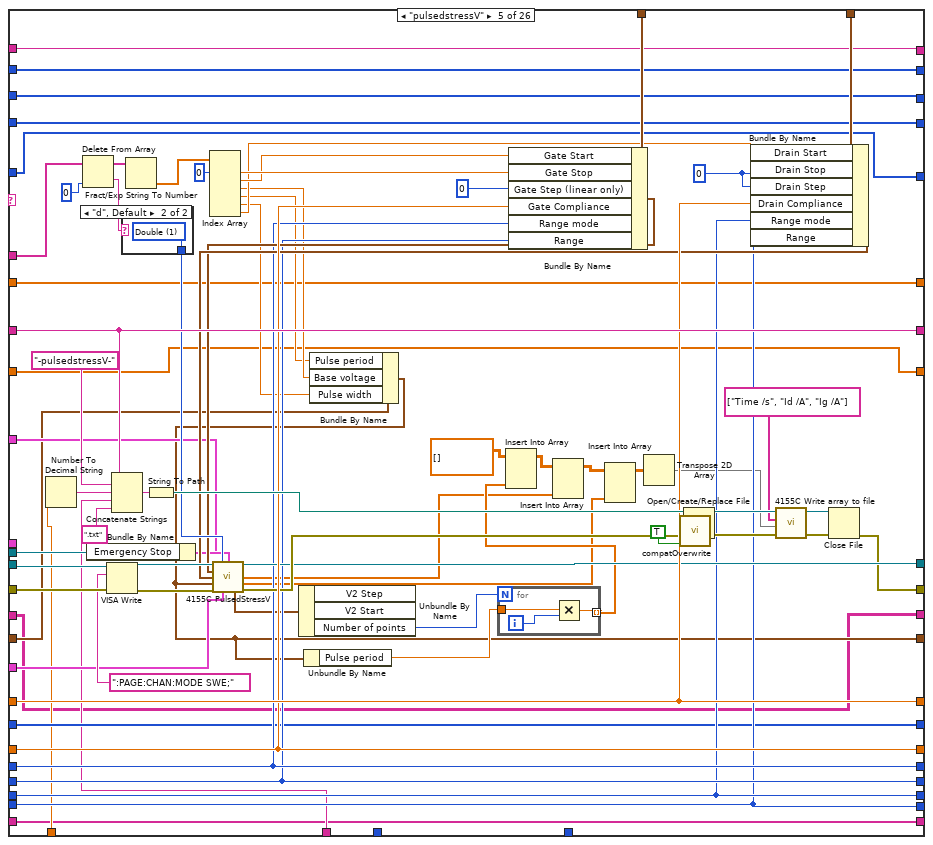
[diagram p10: hidden frame]
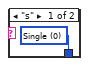
[diagram p11: hidden frame]
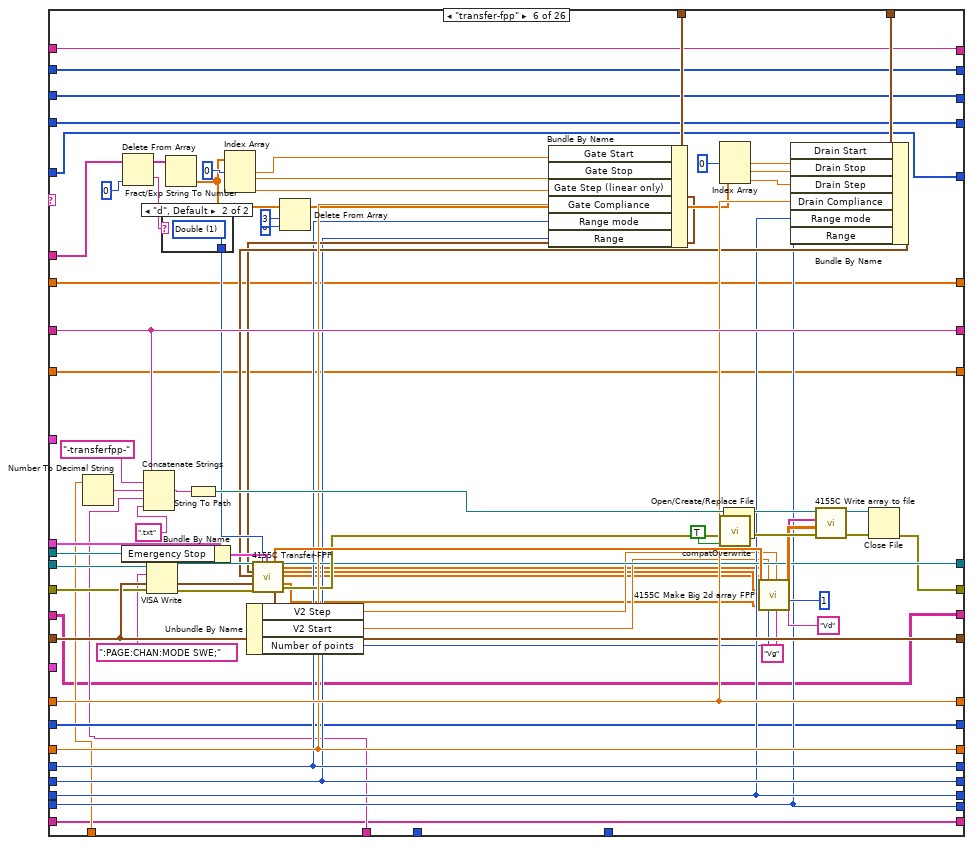
[diagram p12: hidden frame]
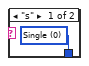
[diagram p13: hidden frame]
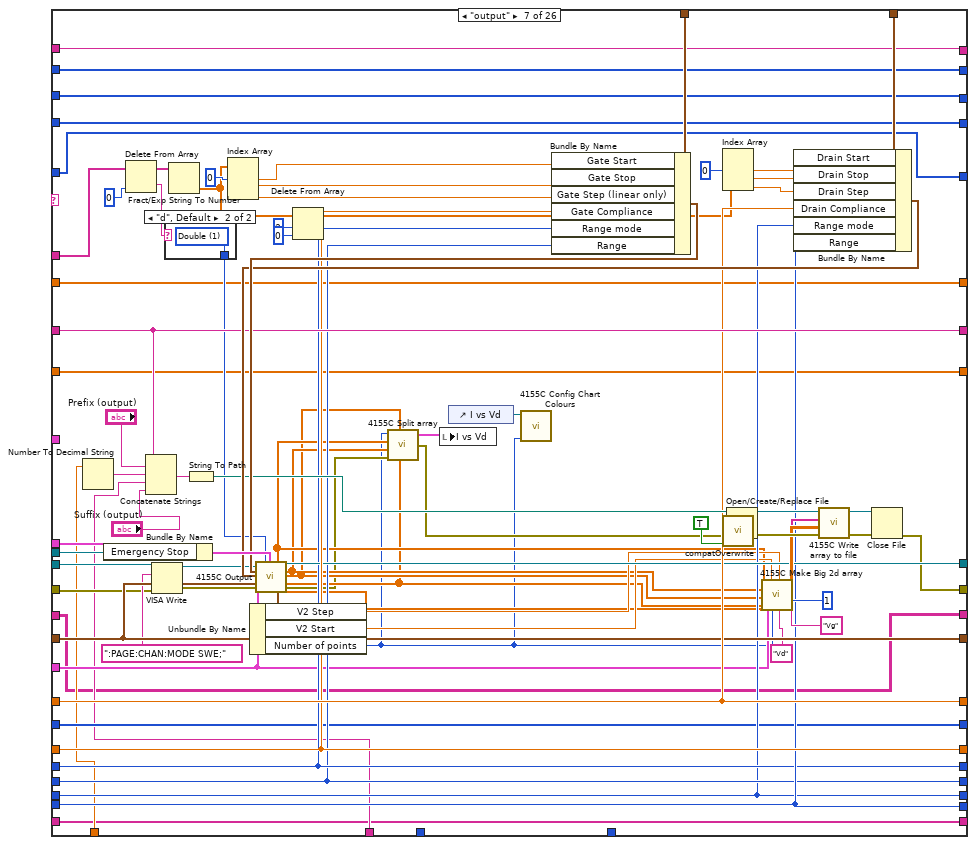
[diagram p14: hidden frame]
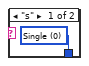
[diagram p15: hidden frame]
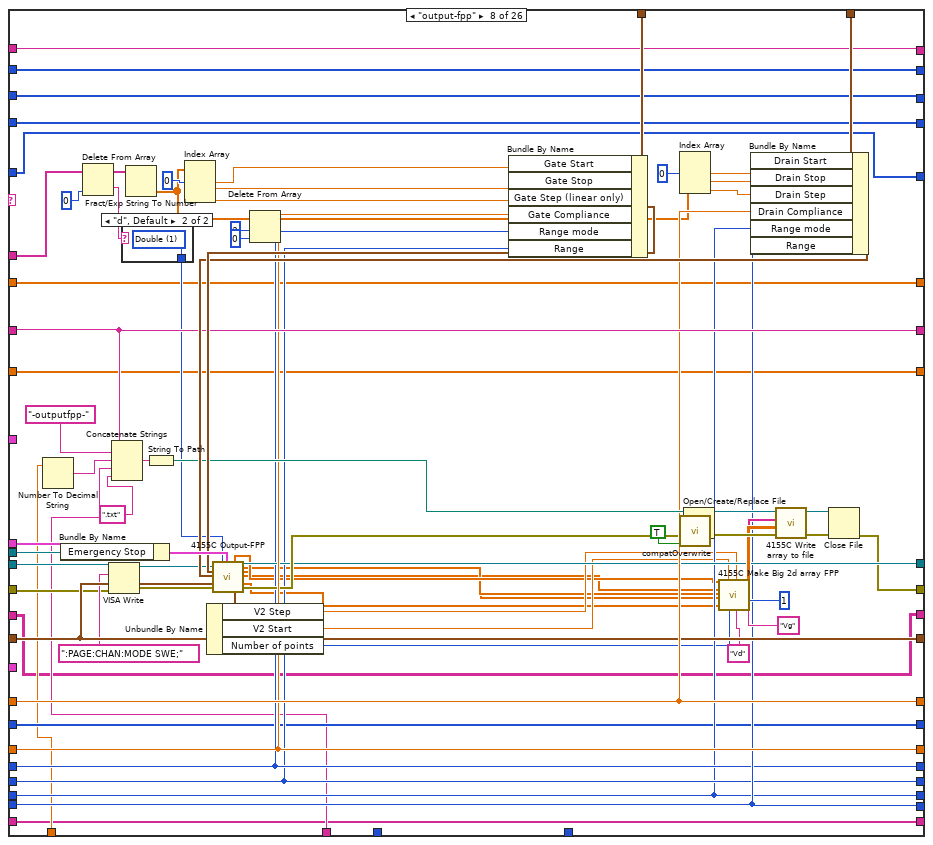
[diagram p16: hidden frame]
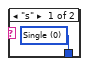
[diagram p17: hidden frame]
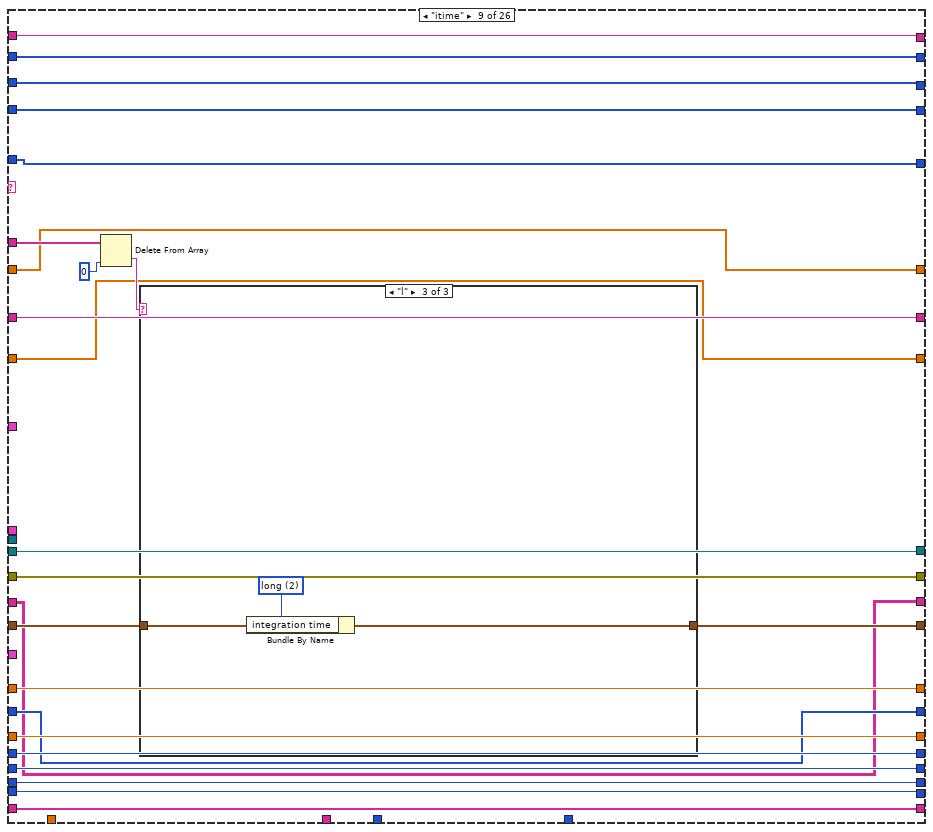
[diagram p18: hidden frame]
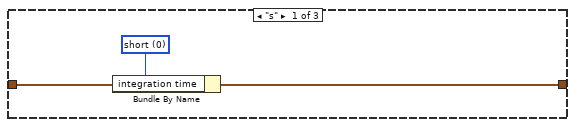
[diagram p19: hidden frame]
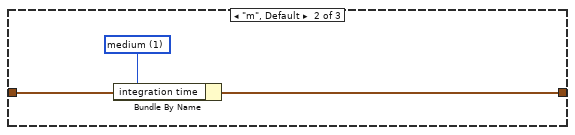
[diagram p20: hidden frame]
diagram:
  w40 = u16 1 items=["Reset All", "Partial reset"] ("Type of reset")
  # "Change from previous version:\n\n- Serial port data are now saved in a table properly."
  # "This is a version specific to the SPM pump."
  # "I add 1 to both the \"total lines\" and the \"line running\" indicators because i and N begin from 0, and the script lines begin from 1."
  # "Bugs:\n\n- Graphs of max and min drain current vs time do not auto-reset between runs. To clear the data you need to restart the vi.\n\n- Do not connect the error message of the Split block if there are unconnected terminals! It will halt the program."
  # "Array size"
  # "%s option converts a spreadsheet string to an array of strings."
  # "0: No of rows of array\n1: No of cols"
  # "Dimitrios Simatos\nv. 5.0"
  # "Changes from original textcontrol.vi:\n\n- Timestamp appears in filename.\n- (Only) transfer and output curves are plotted.\n- Communication with serial port.\n- Can execute any command, as all pattern matching functions were replaced. Previously, commands with special LabVIEW characters could not be executed.\n- Replaced write to file function with write to text file.\n- Replaced while loop with for loop.\n- Replaced 4155C \"Save File\" function and now the vi can save time-dependent variables.\n- Added clock with start time control and various units.\n- Changed filepath in which the program is saved.\n- Added a serial output log that keeps a history.\n- Tab control.\n- Addition of specialized serial read/write file for the SPM OEM pump.\n- Added halt and hard stop."
  # "Search and replace LF with EOL"
  n1 = Equal?(x="integration time", y=u32 0) -> (x = y?=w44:bool)
  n2 = Select(t="Integration time (short)", s=w44, f="Integration time (long)") -> (s? t:f=w48:dbl)
  n3 = call "4155C Get Filename.vi"("error in (no error)"=errorcluster {"status"=FALSE, "code"=0, "source"=""}) -> ("error out"=w35:errorcluster, "path"=w10:path)  [unwired: 2 in, 1 out]
  "Path" <- w10
  n4 = Bundle By Name(cluster="Timings 2", "integration time"="integration time", "Short/Long integration time"=w48, "hold time (sec)"="hold time /s", "delay time (sec)"="delay time /s", "Step Time (0 disables)"="Step delay /s") -> (w33:T6)
  n5 = Path To String(path=w10) -> (string=w11:string)
  n6 = Search and Replace String(replace all?=TRUE ("replace all? (F)"), input string="Program", search string="\n", replace string="\r\n") -> (result string=w23:string)  [unwired: 4 in, 3 out]
  n7 = Match Pattern(string=w11, regular expression=".txt") -> (before substring=w5:string)  [unwired: 1 in, 3 out]
  n8 = Concatenate Strings(w5, "Prefix (script)", ".txt" ("regular expression")) -> (w4:string)
  n9 = call "4155C Initialise.vi"("VISA resource name in"=refnum<visa-resource-name> "GPIB0::14::INSTR", "Reset"="Full Reset", "Type of reset"=w40, "error in (no error)"=w35, "VISA Timeout Value"=u32 10000) -> ("VISA Resource Name out"=w34:refnum<visa-resource-name>, "error out"=w2:errorcluster)
  n10 = Spreadsheet String To Array(delimiter (Tab)="\r\n", format string="%s", spreadsheet string="Program", array type (2D Dbl)="") -> (array=w14:string[][])
  n11 = Array Size(array=w14) -> (size(s)=w18:i32[])
  n12 = String To Path(string=w4) -> (path=w3:path)
  n13 = Write to Text File(file (use dialog)=w3, text=w23, error in=w2) -> (error out=w1:errorcluster)  [unwired: 1 in, 2 out]
  n14 = Index Array(array=w18, index=0) -> (element=w16:i32)
  n15 = for {
    N: w16 -> [w125]
    tunnel: "SMU4" -> [w166]
    shift-left: "Source/Drain Range" -> [w171]
    shift-right: [w167] -> _
    shift-left: "Source/Drain\nRange mode" -> [w172]
    shift-right: [w168] -> _
    shift-left: "Gate Range" -> [w173]
    shift-right: [w169] -> _
    shift-left: "Gate Range\nmode" -> [w174]
    shift-right: [w170] -> _
    shift-left: "Gate: Compliance" -> [w183]
    shift-right: [w179] -> _
    shift-left: "Drain: Compliance" -> [w184]
    shift-right: [w180] -> _
    shift-left: w33 -> [w185]
    shift-right: [w181] -> _
    shift-left: w1 -> [w186]
    shift-right: [w65] -> w9
    shift-left: w34 -> [w187]
    shift-right: [w182] -> _
    shift-left: w5 -> [w188]
    shift-right: [w69] -> _
    tunnel: "Panel Controls 2" -> [w165]
    shift-right: [w136] -> _
    shift-left: _ -> [w164]
    shift-right: [w91] -> _
    shift-left: _ -> [w160]
    tunnel: w14 -> [w159] mode=indexing
    shift-right: [w131] -> _
    shift-left: _ -> [w132]
    shift-right: [w59] -> _
    shift-left: _ -> [w117]
    shift-right: [w92] -> _
    shift-left: _ -> [w110]
    shift-right: [w71] -> _
    shift-left: _ -> [w109]
    shift-right: [w108] -> _
    shift-left: _ -> [w107]
    shift-right: [w64] -> _
    shift-left: _ -> [w88]
    shift-right: [w63] -> _
    shift-left: _ -> [w70]
    shift-right: [w60] -> _
    shift-left: _ -> [w62]
    i -> [w120]
    w50 = "Time /Minutes" ("element")
    # "Serial port data (string)"
    # "Serial port data (table)"
    # "Time array for valve position"
    # "Time array for absolute plunger position"
    # "Valve position"
    # "Pump status"
    # "Absolute plunger position"
    # "Serial port data"
    # "For loop counter"
    # "<-----Equivalent to the 4155C \"Write\" subvi.----->"
    # "Headers"
    # "Save transfer curves in file."
    # "Filepath and name"
    # "Save time-dependent data."
    # "Use the time offset if your measurements do not start at t=0."
    # "Time for Idmax-Idmin"
    # "Rest of elements of command"
    # "Id min"
    # "Id max"
    # "Limit of command arguments (array columns). Raise if needed."
    # "First element of command\n(case select)"
    n16 = Add(x=w125, y=1) -> (x+y=→"Total lines":i32)
    n17 = Add(x=w120, y=1) -> (x+y=→"Line running":i32)
    n18 = Index Array(array=w159, index=0 ("line index")) -> (element=w154:string)
    "Command running:" <- w154
    n19 = Spreadsheet String To Array(delimiter (Tab)=" ", format string="%s", spreadsheet string=w154, array type (2D Dbl)=string[] []) -> (array=w151:string[])
    n20 = control-ref of="Interrupt run"() -> (w178:refnum<vi>)
    n21 = Delete From Array(array=w151, index=0) -> (deleted portion=w152:string, array with subset deleted=w150:string[])  [unwired: 1 in]
    n22 = call "Elapsed Time"("Reset"="Reset", "Auto Reset"="Auto Reset") -> ("Elapsed Time (s)"=w161:dbl)  [unwired: 10 in, 7 out]
    n23 = case shown="0, Default" "Units" {
      tunnel: ["_sec" "_min" "_h"] -> w162
      tunnel: [w189 w193 w196] -> w127
      tunnel: w161 -> [w189 w192 w197]
      frame 0, Default {
      }
      frame 1 {
        n24 = Divide(x=w192, y=60.0) -> (x/y=w193:dbl)
      }
      frame 2 {
        n25 = Divide(x=w197, y=3600.0) -> (x/y=w196:dbl)
      }
    }
    n26 = Add(x=w127, y="Time Offset") -> (x+y=w126:dbl)
    n27 = To Long Integer(number=w126) -> (32bit integer=w89:i32)
    "Elapsed Time" <- w89
    n28 = case shown="\"pump\"" w152 {
      tunnel: w150 -> [w223 w250 w276 w359 w431 w508 w591 w669 w715 w749 w784 w817 w846 w868 _ _ w996 w1065 _ w1146 w1198 w1248 w1326 w1396 w1424 w1483]
      tunnel: w188 -> [w218 w246 w274 w366 w438 w516 w598 w677 w704 w738 w776 w810 w840 w861 w888 w938 w974 w1047 w1086 w1133 w1185 w1236 w1320 w1392 w1426 w1485]
      tunnel: w187 -> [w217 w245 w265 w337 w422 w485 w567 w645 w705 w739 w777 w811 w841 w862 w893 w940 w1002 w1071 w1090 w1152 w1204 w1254 w1332 w1350 w1430 w1489]
      tunnel: w186 -> [w216 w244 w264 w336 w421 w484 w564 w642 w706 w740 w778 w812 w842 w863 w892 w911 w1001 w1070 w1089 w1151 w1203 w1253 w1331 w1349 w1429 w1488]
      tunnel: w185 -> [w215 w243 w273 w362 w397 w512 w594 w673 w714 w748 w775 w809 w839 w860 w891 w935 w965 w1039 w1095 w1126 w1178 w1229 w1319 w1391 w1431 w1490]
      tunnel: w184 -> [w214 w242 w272 w364 w436 w514 w596 w675 w713 w747 w783 w816 w845 w867 w890 w920 w1000 w1069 w1098 w1150 w1202 w1252 w1330 w1400 w1432 w1491]
      tunnel: w183 -> [w213 w241 w271 w363 w435 w513 w595 w674 w712 w746 w782 w815 w844 w866 w889 w921 w975 w1048 w1097 w1134 w1186 w1237 w1321 w1393 w1434 w1492]
      tunnel: [w217 w245 w263 w361 w433 w510 w593 w671 w705 w739 w777 w811 w841 w862 w893 w940 w966 w1021 w1088 w1127 w1179 w1230 w1272 w1352 w1430 w1489] -> w182
      tunnel: [w216 w244 w262 w360 w432 w509 w592 w670 w706 w740 w778 w812 w842 w863 w892 w910 w976 w1022 w1087 w1135 w1187 w1238 w1271 w1351 w1428 w1487] -> w87
      tunnel: [w215 w243 w273 w362 w393 w512 w594 w673 w707 w741 w775 w809 w839 w860 w891 w935 w965 w1039 w1095 w1126 w1178 w1229 w1319 w1391 w1431 w1490] -> w181
      tunnel: [w214 w242 w272 w364 w436 w514 w596 w675 w713 w747 w783 w816 w845 w867 w890 w920 w1000 w1069 w1098 w1150 w1202 w1252 w1330 w1400 w1432 w1491] -> w180
      tunnel: [w213 w241 w271 w363 w435 w513 w595 w674 w712 w746 w782 w815 w844 w866 w889 w921 w975 w1048 w1097 w1134 w1186 w1237 w1321 w1393 w1434 w1492] -> w179
      tunnel: [w218 w246 w274 w366 w438 w516 w598 w677 w704 w738 w776 w810 w840 w861 w888 w938 w974 w1047 w1086 w1133 w1185 w1236 w1320 w1392 w1426 w1485] -> w69
      tunnel: w178 -> [_ _ _ w369 w442 w521 w602 w681 _ _ _ _ _ _ _ _ w971 w1044 _ w1132 w1184 w1235 w1292 w1368 _ _]
      tunnel: "Gate" -> [_ _ _ w346 w425 w495 w578 w656 _ _ _ _ _ _ _ _ _ _ _ _ _ _ _ _ _ _]
      tunnel: "Drain 2" -> [_ _ _ w345 w424 w494 w577 w655 _ _ _ _ _ _ _ _ _ _ _ _ _ _ _ _ _ _]
      tunnel: "Panel Controls" -> [_ _ _ _ _ w493 w576 w654 _ _ _ _ _ _ _ _ _ _ _ _ _ _ _ _ _ _]
      tunnel: w174 -> [w212 w240 w270 w330 w415 w478 w562 w640 w711 w745 _ w808 w838 w859 w887 w922 w961 w1035 w1091 w1122 w1174 w1225 w1315 w1387 w1435 w1493]
      tunnel: w173 -> [w211 w239 w269 w329 w414 w477 w561 w639 w710 w744 w781 _ w829 w865 w886 w923 w962 w1036 w1092 w1123 w1175 w1226 w1316 w1388 w1436 w1494]
      tunnel: w172 -> [w210 w238 w268 w328 w413 w476 w560 w638 w709 w743 w780 w814 w843 _ w885 w924 w963 w1037 w1093 w1124 w1176 w1227 w1317 w1389 w1437 w1495]
      tunnel: w171 -> [w209 w237 w267 w327 w412 w475 w563 w641 w708 w742 w779 w813 _ w864 w884 w925 w964 w1038 w1094 w1125 w1177 w1228 w1318 w1390 w1438 w1496]
      tunnel: [w212 w240 w270 w330 w415 w478 w562 w640 w711 w745 w774 w808 w838 w859 w887 w922 w961 w1035 w1091 w1122 w1174 w1225 w1315 w1387 w1435 w1493] -> w170
      tunnel: [w211 w239 w269 w329 w414 w477 w561 w639 w710 w744 w781 w800 w829 w865 w886 w923 w962 w1036 w1092 w1123 w1175 w1226 w1316 w1388 w1436 w1494] -> w169
      tunnel: [w210 w238 w268 w328 w413 w476 w560 w638 w709 w743 w780 w814 w843 w858 w885 w924 w963 w1037 w1093 w1124 w1176 w1227 w1317 w1389 w1437 w1495] -> w168
      tunnel: [w209 w237 w267 w327 w412 w475 w563 w641 w708 w742 w779 w813 w830 w864 w884 w925 w964 w1038 w1094 w1125 w1177 w1228 w1318 w1390 w1438 w1496] -> w167
      tunnel: w166 -> [_ _ _ w322 w409 _ w556 _ _ _ _ _ _ _ _ _ _ _ _ _ _ _ _ _ _ _]
      tunnel: w165 -> [_ _ _ w320 w408 _ _ _ _ _ _ _ _ _ _ _ _ _ _ _ _ _ _ _ _ _]
      tunnel: [w208 w233 w260 w297 w385 w465 w553 w627 w703 w736 w773 w799 w828 w857 w883 w906 w953 w1019 w1085 w1111 w1167 w1219 w1269 w1345 w1427 w1486] -> w136
      tunnel: w164 -> [w208 w233 w260 w311 w385 w465 w553 w627 w703 w736 w773 w799 w828 w857 w883 w906 w953 w1019 w1085 w1111 w1167 w1219 w1269 w1345 w1427 w1486]
      tunnel: w126 -> [_ _ _ w307 w382 w463 w550 w624 _ _ _ _ _ _ _ w904 w951 w1016 _ w1108 w1164 w1216 w1266 w1341 _ _]
      tunnel: w162 -> [_ _ _ w304 w381 w461 w549 w623 _ _ _ _ _ _ _ w902 w949 w1015 _ w1107 w1163 w1215 w1265 w1342 _ w1454]
      tunnel: w89 -> [_ _ _ w298 _ _ _ _ _ _ _ _ _ _ _ _ _ _ _ _ _ _ _ _ _ w1457]
      tunnel: [w207 w232 w259 w295 w384 w464 w552 w626 w702 w735 w772 w798 w827 w856 w882 w905 w952 w1018 w1084 w1110 w1166 w1218 w1268 w1344 w1433 w1466] -> w91
      tunnel: w160 -> [w207 w232 w259 w303 w384 w464 w552 w626 w702 w735 w772 w798 w827 w856 w882 w905 w952 w1018 w1084 w1110 w1166 w1218 w1268 w1344 w1433 w1466]
      tunnel: [w206 w231 w258 w293 w380 w460 w548 w622 w701 w734 w771 w797 w826 w855 w881 w901 w948 w1014 w1083 w1106 w1162 w1214 w1264 w1340 w1422 w1482] -> w131
      tunnel: w132 -> [w206 w231 w258 w292 w380 w460 w548 w622 w701 w734 w771 w797 w826 w855 w881 w901 w948 w1014 w1083 w1106 w1162 w1214 w1264 w1340 w1422 w1482]
      tunnel: [w205 w230 w257 w285 w379 w459 w538 w621 w700 w733 w770 w796 w825 w854 w880 w900 w947 w1013 w1082 w1105 w1161 w1213 w1263 w1339 w1421 w1481] -> w59
      tunnel: w117 -> [w205 w230 w257 w285 w379 w459 w538 w621 w700 w733 w770 w796 w825 w854 w880 w900 w947 w1013 w1082 w1105 w1161 w1213 w1263 w1339 w1420 w1455]
      tunnel: [w204 w229 w256 w284 w378 w458 w537 w620 w699 w732 w769 w795 w824 w853 w879 w899 w946 w1012 w1081 w1104 w1160 w1212 w1262 w1338 w1406 w1468] -> w92
      tunnel: w110 -> [w204 w229 w256 w284 w378 w458 w537 w620 w699 w732 w769 w795 w824 w853 w879 w899 w946 w1012 w1081 w1104 w1160 w1212 w1262 w1338 w1406 w1467]
      tunnel: [w203 w228 w255 w283 w377 w457 w536 w619 w698 w731 w768 w794 w823 w852 w878 w898 w945 w1011 w1080 w1103 w1159 w1211 w1261 w1337 w1405 w1450] -> w71
      tunnel: w109 -> [w203 w228 w255 w283 w377 w457 w536 w619 w698 w731 w768 w794 w823 w852 w878 w898 w945 w1011 w1080 w1103 w1159 w1211 w1261 w1337 w1405 w1448]
      tunnel: [w202 w227 w254 w282 w376 w456 w535 w618 w697 w730 w767 w793 w822 w851 w877 w897 w944 w1010 w1079 w1102 w1158 w1210 w1260 w1336 w1404 w1447] -> w108
      tunnel: w107 -> [w202 w227 w254 w282 w376 w456 w535 w618 w697 w730 w767 w793 w822 w851 w877 w897 w944 w1010 w1079 w1102 w1158 w1210 w1260 w1336 w1404 w1458]
      tunnel: w89 -> [_ _ _ _ _ _ _ _ _ _ _ _ _ _ _ _ _ _ _ _ _ _ _ _ _ w1446]
      tunnel: w88 -> [w201 w226 w253 w281 w375 w455 w534 w617 w696 w729 w766 w792 w821 w850 w876 w896 w943 w1009 w1078 w1101 w1157 w1209 w1259 w1335 w1403 w1445]
      tunnel: [w201 w226 w253 w281 w375 w455 w534 w617 w696 w729 w766 w792 w821 w850 w876 w896 w943 w1009 w1078 w1101 w1157 w1209 w1259 w1335 w1403 w1444] -> w64
      tunnel: [w200 w225 w252 w280 w374 w454 w533 w616 w695 w728 w765 w791 w820 w849 w875 w895 w942 w1008 w1077 w1100 w1156 w1208 w1258 w1334 w1402 w1443] -> w63
      tunnel: w70 -> [w200 w225 w252 w280 w374 w454 w533 w616 w695 w728 w765 w791 w820 w849 w875 w895 w942 w1008 w1077 w1100 w1156 w1208 w1258 w1334 w1402 w1442]
      tunnel: [w199 w224 w251 w279 w373 w453 w532 w615 w694 w727 w764 w790 w819 w848 w874 w894 w941 w1007 w1076 w1099 w1155 w1207 w1257 w1333 w1401 w1440] -> w60
      tunnel: w62 -> [w199 w224 w251 w279 w373 w453 w532 w615 w694 w727 w764 w790 w819 w848 w874 w894 w941 w1007 w1076 w1099 w1155 w1207 w1257 w1333 w1401 w1439]
      frame "wait" {
        n29 = Index Array(array=w223, index=0 ("Index")) -> (element=w221:string)
        n30 = Decimal String To Number(string=w221, default (0L)=u32 0) -> (number=w220:u32)  [unwired: 1 in, 1 out]
        n31 = Wait (ms)(milliseconds to wait=w220) -> ()  [unwired: 1 out]
      }
      frame "wait-min" {
        n32 = Index Array(array=w250, index=0 ("Index")) -> (element=w248:string)
        n33 = Decimal String To Number(string=w248, default (0L)=u32 0) -> (number=w236:u32)  [unwired: 1 in, 1 out]
        n34 = Multiply(x=w236, y=u32 60000) -> (x*y=w235:u32)
        n35 = Wait (ms)(milliseconds to wait=w235) -> ()  [unwired: 1 out]
      }
      frame "standby" {
        n36 = Index Array(array=w276, index=0 ("Index")) -> (element=w266:string)
        n37 = case shown="\"on\"" w266 {
          tunnel: [":PAGE:SCON:STAN 0" ":PAGE:SCON:STAN 1"] -> w261
          frame "off", Default {
          }
          frame "on" {
          }
        }
        n38 = VISA Write(VISA resource name=w265, write buffer=w261, error in (no error)=w264) -> (VISA resource name out=w263:refnum<visa-resource-name>, error out=w262:errorcluster)  [unwired: 1 out]
      }
      frame "transfer" {
        # "Don't connect the error lines\nof the two Split blocks!"
        # "Adjusts graph colors."
        # "Time array"
        n39 = Bundle By Name(cluster=w320, "Emergency Stop"=w369) -> (w321:T2)
        n40 = Number To Decimal String(number=w307) -> (decimal integer string=w306:string)  [unwired: 1 in]
        n41 = Delete From Array(array=w359, index=0 ("Index")) -> (deleted portion=w357:string, array with subset deleted=w356:string[])  [unwired: 1 in]
        n42 = Concatenate Strings(w366, "Prefix (transfer)", w306, w304, "Suffix (transfer)") -> (w368:string)
        n43 = VISA Write(VISA resource name=w337, write buffer=":PAGE:CHAN:MODE SWE;" ("write buffer (\"\")"), error in (no error)=w336) -> (VISA resource name out=w334:refnum<visa-resource-name>, error out=w335:errorcluster)  [unwired: 1 out]
        n44 = case shown="\"d\", Default" w357 {
          tunnel: [w371 w372] -> w355
          frame "s" {
            w371 = u16 0 items=["Single", "Double"] ("sweep mode")
          }
          frame "d", Default {
            w372 = u16 1 items=["Single", "Double"] ("sweep mode")
          }
        }
        n45 = String To Path(string=w368) -> (path=w365:path)
        n46 = Fract/Exp String To Number(string=w356) -> (number=w341:dbl[])  [unwired: 3 in, 1 out]
        n47 = Index Array(array=w341, index #1=0 ("Index")) -> (element #1=w354:dbl, element #2=w353:dbl, element #3=w352:dbl)  [unwired: 2 in]
        n48 = Delete From Array(array=w341, length=3 ("Length"), index=0 ("Index")) -> (array with subset deleted=w339:dbl[])  [unwired: 1 out]
        n49 = Build Array (concatenate)(w303, w298) -> (w295:i32[])
        n50 = Bundle By Name(cluster=w346, "Gate Start"=w354, "Gate Stop"=w353, "Gate Step (linear only)"=w352, "Gate Compliance"=w363, "Range mode"=w330, "Range"=w329) -> (w331:T4)
        n51 = call "4155C Split array.vi"("X data in"=w295, "Y1 data in"=w292) -> ("Array of clusters"=w296:cluster{"Y data in":dbl[], "X data in":dbl[]}[])  [unwired: 5 in, 1 out]
        n52 = local write "Id min vs time"(w296) -> ()
        n53 = Index Array(array=w339, index #1=0 ("Index")) -> (element #1=w349:dbl, element #2=w348:dbl, element #3=w347:dbl)  [unwired: 2 in]
        n54 = call <vilib>:"compatOverwrite.vi"("overwrite (F)"=TRUE) -> ("overwrite?"=w319:T7)
        n55 = control-ref of="I vs Vg"() -> (w308:refnum<vi>)
        n56 = Bundle By Name(cluster=w345, "Drain Start"=w349, "Drain Stop"=w348, "Drain Step"=w347, "Drain Compliance"=w364, "Range mode"=w328, "Range"=w327) -> (w332:T5)
        n57 = call "4155C Transfer.vi"("VISA resource name in"=w334, "Gate"=w331, "Drain"=w332, "Timings"=w362, "error in (no error)"=w335, "SMU4"=w322, "sweep mode"=w355, "Panel Controls"=w321) -> ("VG"=w312:dbl[], "Outparams"=w326:T8, "VISA Resource Name out"=w361:refnum<visa-resource-name>, "IS"=w313:dbl[], "ID"=w318:dbl[], "IG"=w314:dbl[], "error out"=w299:errorcluster, "SMU4"=w323:dbl[])  [unwired: 12 in]
        n58 = Unbundle By Name(w326) -> ("V2 Step"=w325:dbl, "V2 Start"=w324:dbl, "Number of points"=w309:i32)
        n59 = call "4155C Split array.vi"("Number of VAR2 steps"=w309, "Y2 data in"=w318, "X data in"=w312, "Y1 data in"=w313, "Y3 data in"=w314, "error in (no error)"=w299) -> ("Array of clusters"=w302:cluster{"Y data in":dbl[], "X data in":dbl[]}[], "error out"=w300:errorcluster)  [unwired: 1 in]
        n60 = local write "I vs Vg"(w302) -> ()
        n61 = Absolute Value(x=w313) -> (abs(x)=w317:dbl[])
        n62 = Array Max & Min(array=w313) -> (max value=w315:dbl)  [unwired: 3 out]
        n63 = Array Max & Min(array=w314) -> (max value=w316:dbl)  [unwired: 3 out]
        n64 = local write "Is"(w315) -> ()
        n65 = Array Max & Min(array=w317) -> (max value=w310:dbl, min value=w294:dbl)  [unwired: 2 out]
        n66 = local write "Ig"(w316) -> ()
        n67 = Build Array (concatenate)(w311, w310) -> (w297:dbl[])
        n68 = call "4155C Split array.vi"("X data in"=w295, "Y1 data in"=w297) -> ("Array of clusters"=w301:cluster{"Y data in":dbl[], "X data in":dbl[]}[])  [unwired: 5 in, 1 out]
        n69 = local write "Id max vs time"(w301) -> ()
        n70 = local write "Id"(w310) -> ()
        n71 = Open/Create/Replace File(file path (use dialog)=w365, error in=w300, operation (0:open)=w319) -> (refnum out=w290:refnum<file>, error out=w288:errorcluster)  [unwired: 3 in, 1 out]
        n72 = call "4155C Make Big 2d array.vi"("1D Var1"=w312, "1d IS"=w313, "1d ID"=w318, "1d IG"=w314, "1d SMU4"=w323, "SMU4"=w322, "VAR2 START"=w324, "Number of VAR2 steps"=w309, "VAR2 STEP"=w325, "VAR1 Name"="Vg", "Decimal places in header"=i8 1, "VAR2 Name"="Vd") -> ("Header array"=w291:string[], "Data array"=w289:dbl[][])  [unwired: 14 in]
        n73 = call "4155C Config Chart Colours.vi"("Numeric"=w309, "XY Graph 2"=w308) -> ()  [unwired: 6 in]
        n74 = call "4155C Write array to file.vi"("Byte Stream File Refnum"=w290, "Header"=w291, "Data Array"=w289, "error in (no error)"=w288) -> ("dup refnum"=w287:refnum<file>, "error out"=w286:errorcluster)  [unwired: 1 in]
        n75 = Build Array (concatenate)(w292, w294) -> (w293:dbl[])
        n76 = Close File(refnum=w287, error in=w286) -> (error out=w360:errorcluster)  [unwired: 1 out]
      }
      frame "pulsedstressV" {
        w391 = 0
        n77 = Number To Decimal String(number=w382) -> (decimal integer string=w439:string)  [unwired: 1 in]
        n78 = Delete From Array(array=w431, index=0 ("Index")) -> (deleted portion=w429:string, array with subset deleted=w428:string[])  [unwired: 1 in]
        n79 = Bundle By Name(cluster=w408, "Emergency Stop"=w442) -> (w410:T2)
        n80 = VISA Write(VISA resource name=w422, write buffer=":PAGE:CHAN:MODE SWE;" ("write buffer (\"\")"), error in (no error)=w421) -> (VISA resource name out=w419:refnum<visa-resource-name>, error out=w420:errorcluster)  [unwired: 1 out]
        n81 = Concatenate Strings(w438, "-pulsedstressV-" ("Substring"), w439, w381, ".txt" ("Substring")) -> (w441:string)
        n82 = case shown="\"d\", Default" w429 {
          tunnel: [w451 w452] -> w427
          frame "s" {
            w451 = u16 0 items=["Single", "Double"] ("sweep mode")
          }
          frame "d", Default {
            w452 = u16 1 items=["Single", "Double"] ("sweep mode")
          }
        }
        n83 = Fract/Exp String To Number(string=w428) -> (number=w423:dbl[])  [unwired: 3 in, 1 out]
        n84 = String To Path(string=w441) -> (path=w437:path)
        n85 = Index Array(array=w423, index #1=0 ("Index")) -> (element #1=w400:dbl, element #2=w399:dbl, element #3=w396:dbl, element #4=w395:dbl, element #5=w394:dbl, element #6=w398:dbl)  [unwired: 5 in]
        n86 = Bundle By Name(cluster=w397, "Pulse period"=w395, "Base voltage"=w396, "Pulse width"=w394) -> (w393:T6)
        n87 = Unbundle By Name(w393) -> ("Pulse period"=w401:dbl)
        n88 = Bundle By Name(cluster=w425, "Gate Start"=w399, "Gate Stop"=w400, "Gate Step (linear only)"=0, "Gate Compliance"=w435, "Range mode"=w415, "Range"=w414) -> (w416:T4)
        n89 = call <vilib>:"compatOverwrite.vi"("overwrite (F)"=TRUE) -> ("overwrite?"=w386:T7)
        n90 = Bundle By Name(cluster=w424, "Drain Start"=w398, "Drain Stop"=w391, "Drain Step"=w391, "Drain Compliance"=w436, "Range mode"=w413, "Range"=w412) -> (w417:T5)
        n91 = call "4155C PulsedStressV.vi"("VISA resource name in"=w419, "sweep mode"=w427, "Panel Controls"=w410, "Gate"=w416, "Drain"=w417, "Timings"=w393, "error in (no error)"=w420, "SMU4"=w409) -> ("VISA Resource Name out"=w433:refnum<visa-resource-name>, "ID"=w389:dbl[], "IG"=w387:dbl[], "Outparams"=w411:T8, "error out"=w434:errorcluster)  [unwired: 3 in]
        n92 = Unbundle By Name(w411) -> ("Number of points"=w388:i32)  [unwired: 2 out]
        n93 = for {
          N: w388 -> [_]
          tunnel: [w448] -> w390 mode=indexing
          tunnel: w401 -> [w450]
          i -> [w449]
          n94 = Multiply(x=w450, y=w449) -> (x*y=w448:dbl)
        }
        n95 = Insert Into Array(array=dbl[][] [] ("Input Array"), new element=w390) -> (w402:dbl[][])  [unwired: 2 in]
        n96 = Insert Into Array(array=w402, new element=w389) -> (w407:dbl[][])  [unwired: 2 in]
        n97 = Insert Into Array(array=w407, new element=w387) -> (w406:dbl[][])  [unwired: 2 in]
        n98 = Transpose 2D Array(2D array=w406) -> (transposed array=w405:dbl[][])
        n99 = Open/Create/Replace File(file path (use dialog)=w437, error in=w434, operation (0:open)=w386) -> (refnum out=w445:refnum<file>, error out=w446:errorcluster)  [unwired: 3 in, 1 out]
        n100 = call "4155C Write array to file.vi"("Byte Stream File Refnum"=w445, "Header"=string[] ["Time /s", "Id /A", "Ig /A"], "Data Array"=w405, "error in (no error)"=w446) -> ("dup refnum"=w443:refnum<file>, "error out"=w444:errorcluster)  [unwired: 1 in]
        n101 = Close File(refnum=w443, error in=w444) -> (error out=w432:errorcluster)  [unwired: 1 out]
      }
      frame "transfer-fpp" {
        n102 = Number To Decimal String(number=w463) -> (decimal integer string=w517:string)  [unwired: 1 in]
        n103 = Bundle By Name(cluster=w493, "Emergency Stop"=w521) -> (w529:T1)
        n104 = Delete From Array(array=w508, index=0 ("Index")) -> (deleted portion=w506:string, array with subset deleted=w505:string[])  [unwired: 1 in]
        n105 = Concatenate Strings(w516, "-transferfpp-" ("Substring"), w517, w461, ".txt" ("Substring")) -> (w519:string)
        n106 = VISA Write(VISA resource name=w485, write buffer=":PAGE:CHAN:MODE SWE;" ("write buffer (\"\")"), error in (no error)=w484) -> (VISA resource name out=w482:refnum<visa-resource-name>, error out=w483:errorcluster)  [unwired: 1 out]
        n107 = case shown="\"d\", Default" w506 {
          tunnel: [w530 w531] -> w504
          frame "s" {
            w530 = u16 0 items=["Single", "Double"] ("sweep mode")
          }
          frame "d", Default {
            w531 = u16 1 items=["Single", "Double"] ("sweep mode")
          }
        }
        n108 = Fract/Exp String To Number(string=w505) -> (number=w489:dbl[])  [unwired: 3 in, 1 out]
        n109 = String To Path(string=w519) -> (path=w515:path)
        n110 = Index Array(array=w489, index #1=0 ("Index")) -> (element #1=w503:dbl, element #2=w502:dbl, element #3=w501:dbl)  [unwired: 2 in]
        n111 = Delete From Array(array=w489, length=3 ("Length"), index=0 ("Index")) -> (array with subset deleted=w487:dbl[])  [unwired: 1 out]
        n112 = Bundle By Name(cluster=w495, "Gate Start"=w503, "Gate Stop"=w502, "Gate Step (linear only)"=w501, "Gate Compliance"=w513, "Range mode"=w478, "Range"=w477) -> (w479:T4)
        n113 = Index Array(array=w487, index #1=0 ("Index")) -> (element #1=w498:dbl, element #2=w497:dbl, element #3=w496:dbl)  [unwired: 2 in]
        n114 = call <vilib>:"compatOverwrite.vi"("overwrite (F)"=TRUE) -> ("overwrite?"=w466:T7)
        n115 = Bundle By Name(cluster=w494, "Drain Start"=w498, "Drain Stop"=w497, "Drain Step"=w496, "Drain Compliance"=w514, "Range mode"=w476, "Range"=w475) -> (w480:T5)
        n116 = call "4155C Transfer-FPP.vi"("VISA resource name in"=w482, "Gate"=w479, "Drain"=w480, "Timings"=w512, "error in (no error)"=w483, "sweep mode"=w504, "Panel Controls"=w529) -> ("VG"=w520:dbl[], "Outparams"=w474:T8, "VISA Resource Name out"=w510:refnum<visa-resource-name>, "Vprobe2"=w470:dbl[], "ID"=w469:dbl[], "IG"=w468:dbl[], "Vprobe1"=w467:dbl[], "error out"=w511:errorcluster)  [unwired: 13 in]
        n117 = Unbundle By Name(w474) -> ("V2 Step"=w473:dbl, "V2 Start"=w472:dbl, "Number of points"=w471:i32)
        n118 = Open/Create/Replace File(file path (use dialog)=w515, error in=w511, operation (0:open)=w466) -> (refnum out=w526:refnum<file>, error out=w527:errorcluster)  [unwired: 3 in, 1 out]
        n119 = call "4155C Make Big 2d array FPP.vi"("1D Var1"=w520, "1d ID"=w469, "1d Vp2"=w470, "1d IG"=w468, "1d Vp1"=w467, "VAR2 START"=w472, "Number of VAR2 steps"=w471, "VAR2 STEP"=w473, "VAR1 Name"="Vg", "Decimal places in header"=i8 1, "VAR2 Name"="Vd") -> ("Header array"=w522:string[], "Data array"=w523:dbl[][])  [unwired: 15 in]
        n120 = call "4155C Write array to file.vi"("Byte Stream File Refnum"=w526, "Header"=w522, "Data Array"=w523, "error in (no error)"=w527) -> ("dup refnum"=w524:refnum<file>, "error out"=w525:errorcluster)  [unwired: 1 in]
        n121 = Close File(refnum=w524, error in=w525) -> (error out=w509:errorcluster)  [unwired: 1 out]
      }
      frame "output" {
        n122 = Number To Decimal String(number=w550) -> (decimal integer string=w599:string)  [unwired: 1 in]
        n123 = Bundle By Name(cluster=w576, "Emergency Stop"=w602) -> (w612:T1)
        n124 = Delete From Array(array=w591, index=0 ("Index")) -> (deleted portion=w589:string, array with subset deleted=w588:string[])  [unwired: 1 in]
        n125 = Concatenate Strings(w598, "Prefix (output)", w599, w549, "Suffix (output)") -> (w601:string)
        n126 = VISA Write(VISA resource name=w567, write buffer=":PAGE:CHAN:MODE SWE;" ("write buffer (\"\")"), error in (no error)=w564) -> (VISA resource name out=w566:refnum<visa-resource-name>, error out=w565:errorcluster)  [unwired: 1 out]
        n127 = case shown="\"d\", Default" w589 {
          tunnel: [w613 w614] -> w587
          frame "s" {
            w613 = u16 0 items=["Single", "Double"] ("sweep mode")
          }
          frame "d", Default {
            w614 = u16 1 items=["Single", "Double"] ("sweep mode")
          }
        }
        n128 = Fract/Exp String To Number(string=w588) -> (number=w570:dbl[])  [unwired: 3 in, 1 out]
        n129 = String To Path(string=w601) -> (path=w597:path)
        n130 = Index Array(array=w570, index #1=0 ("Index")) -> (element #1=w586:dbl, element #2=w585:dbl, element #3=w584:dbl)  [unwired: 2 in]
        n131 = Delete From Array(array=w570, length=3 ("Length"), index=0 ("Index")) -> (array with subset deleted=w569:dbl[])  [unwired: 1 out]
        n132 = control-ref of="I vs Vd"() -> (w540:refnum<vi>)
        n133 = Bundle By Name(cluster=w578, "Gate Start"=w586, "Gate Stop"=w585, "Gate Step (linear only)"=w584, "Gate Compliance"=w595, "Range mode"=w562, "Range"=w561) -> (w611:T4)
        n134 = Index Array(array=w569, index #1=0 ("Index")) -> (element #1=w581:dbl, element #2=w580:dbl, element #3=w579:dbl)  [unwired: 2 in]
        n135 = call <vilib>:"compatOverwrite.vi"("overwrite (F)"=TRUE) -> ("overwrite?"=w554:T7)
        n136 = Bundle By Name(cluster=w577, "Drain Start"=w581, "Drain Stop"=w580, "Drain Step"=w579, "Drain Compliance"=w596, "Range mode"=w560, "Range"=w563) -> (w610:T5)
        n137 = call "4155C Output.vi"("VISA resource name in"=w566, "Gate"=w611, "Drain"=w610, "Timings"=w594, "error in (no error)"=w565, "SMU4"=w556, "sweep mode"=w587, "Panel controls"=w612) -> ("VD"=w547:dbl[], "Outparams"=w558:T8, "VISA Resource Name out"=w593:refnum<visa-resource-name>, "IS"=w546:dbl[], "ID"=w545:dbl[], "IG"=w544:dbl[], "error out"=w542:errorcluster, "SMU4"=w555:dbl[])  [unwired: 12 in]
        n138 = Unbundle By Name(w558) -> ("V2 Step"=w559:dbl, "V2 Start"=w557:dbl, "Number of points"=w539:i32)
        n139 = call "4155C Split array.vi"("Number of VAR2 steps"=w539, "Y2 data in"=w545, "X data in"=w547, "Y1 data in"=w546, "Y3 data in"=w544, "error in (no error)"=w542) -> ("Array of clusters"=w543:cluster{"Y data in":dbl[], "X data in":dbl[]}[], "error out"=w541:errorcluster)  [unwired: 1 in]
        n140 = local write "I vs Vd"(w543) -> ()
        n141 = call "4155C Config Chart Colours.vi"("Numeric"=w539, "XY Graph 2"=w540) -> ()  [unwired: 6 in]
        n142 = Open/Create/Replace File(file path (use dialog)=w597, error in=w541, operation (0:open)=w554) -> (refnum out=w607:refnum<file>, error out=w608:errorcluster)  [unwired: 3 in, 1 out]
        n143 = call "4155C Make Big 2d array.vi"("1D Var1"=w547, "1d IS"=w546, "1d ID"=w545, "1d IG"=w544, "1d SMU4"=w555, "SMU4"=w556, "VAR2 START"=w557, "Number of VAR2 steps"=w539, "VAR2 STEP"=w559, "VAR1 Name"="Vd", "Decimal places in header"=i8 1, "VAR2 Name"="Vg") -> ("Header array"=w603:string[], "Data array"=w604:dbl[][])  [unwired: 14 in]
        n144 = call "4155C Write array to file.vi"("Byte Stream File Refnum"=w607, "Header"=w603, "Data Array"=w604, "error in (no error)"=w608) -> ("dup refnum"=w605:refnum<file>, "error out"=w606:errorcluster)  [unwired: 1 in]
        n145 = Close File(refnum=w605, error in=w606) -> (error out=w592:errorcluster)  [unwired: 1 out]
      }
      frame "output-fpp" {
        n146 = Number To Decimal String(number=w624) -> (decimal integer string=w678:string)  [unwired: 1 in]
        n147 = Bundle By Name(cluster=w654, "Emergency Stop"=w681) -> (w691:T1)
        n148 = Delete From Array(array=w669, index=0 ("Index")) -> (deleted portion=w667:string, array with subset deleted=w666:string[])  [unwired: 1 in]
        n149 = VISA Write(VISA resource name=w645, write buffer=":PAGE:CHAN:MODE SWE;" ("write buffer (\"\")"), error in (no error)=w642) -> (VISA resource name out=w644:refnum<visa-resource-name>, error out=w643:errorcluster)  [unwired: 1 out]
        n150 = Concatenate Strings(w677, "-outputfpp-" ("Substring"), w678, w623, ".txt" ("Substring")) -> (w680:string)
        n151 = case shown="\"d\", Default" w667 {
          tunnel: [w692 w693] -> w665
          frame "s" {
            w692 = u16 0 items=["Single", "Double"] ("sweep mode")
          }
          frame "d", Default {
            w693 = u16 1 items=["Single", "Double"] ("sweep mode")
          }
        }
        n152 = Fract/Exp String To Number(string=w666) -> (number=w648:dbl[])  [unwired: 3 in, 1 out]
        n153 = String To Path(string=w680) -> (path=w676:path)
        n154 = Index Array(array=w648, index #1=0 ("Index")) -> (element #1=w664:dbl, element #2=w663:dbl, element #3=w662:dbl)  [unwired: 2 in]
        n155 = Delete From Array(array=w648, length=3 ("Length"), index=0 ("Index")) -> (array with subset deleted=w647:dbl[])  [unwired: 1 out]
        n156 = Bundle By Name(cluster=w656, "Gate Start"=w664, "Gate Stop"=w663, "Gate Step (linear only)"=w662, "Gate Compliance"=w674, "Range mode"=w640, "Range"=w639) -> (w690:T4)
        n157 = Index Array(array=w647, index #1=0 ("Index")) -> (element #1=w659:dbl, element #2=w658:dbl, element #3=w657:dbl)  [unwired: 2 in]
        n158 = call <vilib>:"compatOverwrite.vi"("overwrite (F)"=TRUE) -> ("overwrite?"=w628:T7)
        n159 = Bundle By Name(cluster=w655, "Drain Start"=w659, "Drain Stop"=w658, "Drain Step"=w657, "Drain Compliance"=w675, "Range mode"=w638, "Range"=w641) -> (w689:T5)
        n160 = call "4155C Output-FPP.vi"("VISA resource name in"=w644, "Gate"=w690, "Drain"=w689, "Timings"=w673, "error in (no error)"=w643, "sweep mode"=w665, "Panel controls"=w691) -> ("VD"=w633:dbl[], "Outparams"=w636:T8, "VISA Resource Name out"=w671:refnum<visa-resource-name>, "Vprobe2"=w632:dbl[], "ID"=w631:dbl[], "IG"=w630:dbl[], "Vprobe1"=w629:dbl[], "error out"=w672:errorcluster)  [unwired: 13 in]
        n161 = Unbundle By Name(w636) -> ("V2 Step"=w637:dbl, "V2 Start"=w635:dbl, "Number of points"=w634:i32)
        n162 = Open/Create/Replace File(file path (use dialog)=w676, error in=w672, operation (0:open)=w628) -> (refnum out=w686:refnum<file>, error out=w687:errorcluster)  [unwired: 3 in, 1 out]
        n163 = call "4155C Make Big 2d array FPP.vi"("1D Var1"=w633, "1d ID"=w631, "1d Vp2"=w632, "1d IG"=w630, "1d Vp1"=w629, "VAR2 START"=w635, "Number of VAR2 steps"=w634, "VAR2 STEP"=w637, "VAR1 Name"="Vd", "Decimal places in header"=i8 1, "VAR2 Name"="Vg") -> ("Header array"=w682:string[], "Data array"=w683:dbl[][])  [unwired: 15 in]
        n164 = call "4155C Write array to file.vi"("Byte Stream File Refnum"=w686, "Header"=w682, "Data Array"=w683, "error in (no error)"=w687) -> ("dup refnum"=w684:refnum<file>, "error out"=w685:errorcluster)  [unwired: 1 in]
        n165 = Close File(refnum=w684, error in=w685) -> (error out=w670:errorcluster)  [unwired: 1 out]
      }
      frame "itime" {
        n166 = Delete From Array(array=w715, index=0 ("Index")) -> (deleted portion=w716:string)  [unwired: 1 in, 1 out]
        n167 = case shown="\"l\"" w716 {
          tunnel: w714 -> [w720 w722 w725]
          tunnel: [w719 w721 w724] -> w707
          frame "s" {
            w718 = u32 0 items=["short  ", "medium  ", "long  "] ("integration time 2")
            n168 = Bundle By Name(cluster=w720, "integration time"=w718) -> (w719:T6)
          }
          frame "m", Default {
            w723 = u32 1 items=["short  ", "medium  ", "long  "] ("integration time 2")
            n169 = Bundle By Name(cluster=w722, "integration time"=w723) -> (w721:T6)
          }
          frame "l" {
            w726 = u32 2 items=["short  ", "medium  ", "long  "] ("integration time 2")
            n170 = Bundle By Name(cluster=w725, "integration time"=w726) -> (w724:T6)
          }
        }
      }
      frame "pulsed" {
        n171 = Delete From Array(array=w749, index=0 ("Index")) -> (deleted portion=w750:string, array with subset deleted=w737:string[])  [unwired: 1 in]
        n172 = case shown="\"on\", Default" w750 {
          tunnel: w748 -> [w760 w763]
          tunnel: [w759 w762] -> w741
          tunnel: w737 -> [w757 _]
          frame "on", Default {
            w758 = u16 1 items=["Continuous", "Pulsed"] ("sweep method")
            n173 = Fract/Exp String To Number(string=w757) -> (number=w755:dbl[])  [unwired: 3 in, 1 out]
            n174 = Index Array(array=w755, index #1=0 ("Index")) -> (element #1=w754:dbl, element #2=w753:dbl, element #3=w752:dbl)  [unwired: 2 in]
            n175 = Bundle By Name(cluster=w760, "sweep method"=w758, "Pulse period"=w754, "Base voltage"=w753, "Pulse width"=w752) -> (w759:T6)
          }
          frame "off" {
            w761 = u16 0 items=["Continuous", "Pulsed"] ("sweep method")
            n176 = Bundle By Name(cluster=w763, "sweep method"=w761) -> (w762:T6)
          }
        }
      }
      frame "gaterangemode" {
        n177 = Delete From Array(array=w784, index=0 ("Index")) -> (deleted portion=w785:string)  [unwired: 1 in, 1 out]
        n178 = case shown="\"f\"" w785 {
          tunnel: [w787 w788 w789] -> w774
          frame "a", Default {
            w787 = u16 0 items=["Auto", "Limited", "Fixed"] ("Gate Range\nmode 2")
          }
          frame "f" {
            w788 = u16 2 items=["Auto", "Limited", "Fixed"] ("Gate Range\nmode 2")
          }
          frame "l" {
            w789 = u16 1 items=["Auto", "Limited", "Fixed"] ("Gate Range\nmode 2")
          }
        }
      }
      frame "gaterange" {
        (unwired) u8 11 items=["10fA  ", "100fA  ", "1nA  ", "10nA", "100nA", "1uA", "10uA", "100uA", "1mA", "10mA", "100mA", "1A"] ("Gate Range 2")
        n179 = Delete From Array(array=w817, index=0 ("Index")) -> (deleted portion=w807:string)  [unwired: 1 in, 1 out]
        n180 = Scan Value(string=w807, format string="") -> (value=w805:dbl)  [unwired: 1 in, 1 out]
        n181 = Logarithm Base 10(1:w805) -> (0:w804:dbl)
        n182 = Round To Nearest(number=w804) -> (nearest integer value=w803:dbl)
        n183 = Add(x=w803, y=11.0) -> (x+y=w801:dbl)
        n184 = To Unsigned Byte Integer(number=w801) -> (unsigned 8bit integer=w800:u8)
      }
      frame "drainrange" {
        (unwired) u8 11 items=["10fA  ", "100fA  ", "1nA  ", "10nA", "100nA", "1uA", "10uA", "100uA", "1mA", "10mA", "100mA", "1A"] ("Gate Range 2")
        n185 = Delete From Array(array=w846, index=0 ("Index")) -> (deleted portion=w837:string)  [unwired: 1 in, 1 out]
        n186 = Scan Value(string=w837, format string="") -> (value=w835:dbl)  [unwired: 1 in, 1 out]
        n187 = Logarithm Base 10(1:w835) -> (0:w834:dbl)
        n188 = Round To Nearest(number=w834) -> (nearest integer value=w833:dbl)
        n189 = Add(x=w833, y=11.0) -> (x+y=w831:dbl)
        n190 = To Unsigned Byte Integer(number=w831) -> (unsigned 8bit integer=w830:u8)
      }
      frame "drainrangemode" {
        n191 = Delete From Array(array=w868, index=0 ("Index")) -> (deleted portion=w869:string)  [unwired: 1 in, 1 out]
        n192 = case shown="\"f\"" w869 {
          tunnel: [w871 w872 w873] -> w858
          frame "a", Default {
            w871 = u16 0 items=["Auto", "Limited", "Fixed"] ("Gate Range\nmode 2")
          }
          frame "f" {
            w872 = u16 2 items=["Auto", "Limited", "Fixed"] ("Gate Range\nmode 2")
          }
          frame "l" {
            w873 = u16 1 items=["Auto", "Limited", "Fixed"] ("Gate Range\nmode 2")
          }
        }
      }
      frame "Error", Default {
      }
      frame "logfile" {
        n193 = Number To Decimal String(number=w904) -> (decimal integer string=w939:string)  [unwired: 1 in]
        n194 = Concatenate Strings(w938, "logfile" ("Substring"), w939, w902, ".txt" ("Substring")) -> (w936:string)
        n195 = String To Path(string=w936) -> (path=w909:path)
        n196 = Unbundle(w935) -> ("integration time"=w934:u32, "Short/Long integration time"=w933:dbl, "hold time (sec)"=w932:dbl, "delay time (sec)"=w931:dbl, "Step Time (0 disables)"=w930:dbl, "sweep method"=w929:u16, "Pulse period"=w928:dbl, "Base voltage"=w927:dbl, "Pulse width"=w926:dbl)
        n197 = Build Array(w934, w933, w932, w931, w930, w929, w928, w927, w926, w920, w921, w922, w923, w924, w925) -> (w913:dbl[])
        n198 = Insert Into Array(array=dbl[][] [] ("Input Array"), new element=w913) -> (w912:dbl[][])  [unwired: 2 in]
        n199 = call <vilib>:"compatOverwrite.vi"("overwrite (F)"=TRUE) -> ("overwrite?"=w907:T7)
        n200 = Open/Create/Replace File(file path (use dialog)=w909, error in=w911, operation (0:open)=w907) -> (refnum out=w917:refnum<file>, error out=w916:errorcluster)  [unwired: 3 in, 1 out]
        n201 = call "4155C Write array to file.vi"("Byte Stream File Refnum"=w917, "Header"=string[] ["Int Time", "Short/Long Itime", "Hold time", "Delay time", "Step time", "Sweep method", "Pulse period", "Base Voltage", "Pulse width", "Drain compliance", "Gate compliance", "Gate range mode", "Gate range", "S/D range mode", "S/D range"], "Data Array"=w912, "error in (no error)"=w916) -> ("dup refnum"=w919:refnum<file>, "error out"=w918:errorcluster)  [unwired: 1 in]
        n202 = Close File(refnum=w919, error in=w918) -> (error out=w910:errorcluster)  [unwired: 1 out]
      }
      frame "sample" {
        n203 = Number To Decimal String(number=w951) -> (decimal integer string=w999:string)  [unwired: 1 in]
        n204 = Fract/Exp String To Number(string=w996) -> (number=w957:dbl[])  [unwired: 3 in, 1 out]
        n205 = Concatenate Strings(w974, "-sample-" ("Substring"), w999, w949, ".txt" ("Substring")) -> (w997:string)
        n206 = String To Path(string=w997) -> (path=w978:path)
        n207 = Index Array(array=w957, index=0 ("Index")) -> (element=w994:dbl)
        n208 = Index Array(array=w957, index=2 ("Index")) -> (element=w990:dbl)
        n209 = Index Array(array=w957, index=3 ("Index")) -> (element=w959:dbl)
        n210 = Index Array(array=w957, index=4 ("Index")) -> (element=w956:dbl)
        n211 = call "4155C Config Sampling Measurements.vi"("Sampling interval"=w956, "Sample time"=w959, "Display on/off"=TRUE, "Timings"=w965, "Num Points"=w990, "error in (no error)"=w1001, "Drain Compliance"=w1000, "Gate Compliance"=w975, "VISA session"=w1002) -> ("error out"=w1003:errorcluster, "dup VISA resource name"=w1004:refnum<visa-resource-name>)  [unwired: 1 in]
        n212 = Index Array(array=w957, index=1 ("Index")) -> (element=w991:dbl)
        n213 = call "4155C Take Sample.vi"("Emergency Stop"=w971, "error in (no error)"=w1003, "Vd"=w991, "Vg"=w994, "VISA resource name in"=w1004) -> ("error out"=w969:errorcluster, "Id"=w1006:dbl[], "Ig"=w980:dbl[], "VISA Resource Name out"=w967:refnum<visa-resource-name>, "Is"=w1005:dbl[], "Time"=w984:dbl[])  [unwired: 1 in]
        n214 = Insert Into Array(array=dbl[][] [] ("Input Array"), new element=w984) -> (w983:dbl[][])  [unwired: 2 in]
        n215 = Insert Into Array(array=w983, new element=w980) -> (w982:dbl[][])  [unwired: 2 in]
        n216 = Insert Into Array(array=w982, new element=w1006) -> (w981:dbl[][])  [unwired: 2 in]
        n217 = VISA Write(VISA resource name=w967, write buffer=":DISP ON" ("write buffer (\"\")"), error in (no error)=w969) -> (VISA resource name out=w966:refnum<visa-resource-name>, error out=w968:errorcluster)  [unwired: 1 out]
        n218 = Insert Into Array(array=w981, new element=w1005) -> (w973:dbl[][])  [unwired: 2 in]
        n219 = Transpose 2D Array(2D array=w973) -> (transposed array=w972:dbl[][])
        n220 = call <vilib>:"compatOverwrite.vi"("overwrite (F)"=TRUE) -> ("overwrite?"=w954:T7)
        n221 = Open/Create/Replace File(file path (use dialog)=w978, error in=w968, operation (0:open)=w954) -> (refnum out=w987:refnum<file>, error out=w986:errorcluster)  [unwired: 3 in, 1 out]
        n222 = call "4155C Write array to file.vi"("Byte Stream File Refnum"=w987, "Header"=string[] ["Time /s", "Ig /A", "Id /A", "Is /A"], "Data Array"=w972, "error in (no error)"=w986) -> ("dup refnum"=w989:refnum<file>, "error out"=w988:errorcluster)  [unwired: 1 in]
        n223 = Close File(refnum=w989, error in=w988) -> (error out=w976:errorcluster)  [unwired: 1 out]
      }
      frame "samplei" {
        n224 = Number To Decimal String(number=w1016) -> (decimal integer string=w1068:string)  [unwired: 1 in]
        n225 = Fract/Exp String To Number(string=w1065) -> (number=w1032:dbl[])  [unwired: 3 in, 1 out]
        n226 = Concatenate Strings(w1047, "-samplei-" ("Substring"), w1068, w1015, ".txt" ("Substring")) -> (w1066:string)
        n227 = String To Path(string=w1066) -> (path=w1050:path)
        n228 = Index Array(array=w1032, index=4 ("Index")) -> (element=w1026:dbl)
        n229 = Index Array(array=w1032, index=3 ("Index")) -> (element=w1027:dbl)
        n230 = Index Array(array=w1032, index=1 ("Index")) -> (element=w1029:dbl)
        n231 = Index Array(array=w1032, index=0 ("Index")) -> (element=w1030:dbl)
        n232 = Index Array(array=w1032, index=2 ("Index")) -> (element=w1028:dbl)
        n233 = call "4155C Config SamplingI Measurements.vi"("Sample time"=w1028, "Display on/off"=TRUE, "Timings"=w1039, "Num Points"=w1029, "error in (no error)"=w1070, "Sampling interval"=w1027, "VISA session"=w1071) -> ("error out"=w1072:errorcluster, "dup VISA resource name"=w1073:refnum<visa-resource-name>)  [unwired: 3 in]
        n234 = call "4155C Take SampleI.vi"("Emergency Stop"=w1044, "error in (no error)"=w1072, "Idg 2"=w1030, "Vdg compliance 2"=w1026, "VISA resource name in"=w1073) -> ("error out"=w1042:errorcluster, "Idg"=w1075:dbl[], "Vdg"=w1052:dbl[], "VISA Resource Name out"=w1040:refnum<visa-resource-name>, "Is"=w1074:dbl[], "Time"=w1056:dbl[])  [unwired: 1 in]
        n235 = Insert Into Array(array=dbl[][] [] ("Input Array"), new element=w1056) -> (w1055:dbl[][])  [unwired: 2 in]
        n236 = Insert Into Array(array=w1055, new element=w1052) -> (w1054:dbl[][])  [unwired: 2 in]
        n237 = Insert Into Array(array=w1054, new element=w1075) -> (w1053:dbl[][])  [unwired: 2 in]
        n238 = VISA Write(VISA resource name=w1040, write buffer=":DISP ON" ("write buffer (\"\")"), error in (no error)=w1042) -> (VISA resource name out=w1025:refnum<visa-resource-name>, error out=w1041:errorcluster)  [unwired: 1 out]
        n239 = Insert Into Array(array=w1053, new element=w1074) -> (w1046:dbl[][])  [unwired: 2 in]
        n240 = Transpose 2D Array(2D array=w1046) -> (transposed array=w1045:dbl[][])
        n241 = call <vilib>:"compatOverwrite.vi"("overwrite (F)"=TRUE) -> ("overwrite?"=w1020:T7)
        n242 = Open/Create/Replace File(file path (use dialog)=w1050, error in=w1041, operation (0:open)=w1020) -> (refnum out=w1059:refnum<file>, error out=w1058:errorcluster)  [unwired: 3 in, 1 out]
        n243 = call "4155C Write array to file.vi"("Byte Stream File Refnum"=w1059, "Header"=string[] ["Time /s", "Vdg /V", "Idg /A", "Is /A"], "Data Array"=w1045, "error in (no error)"=w1058) -> ("dup refnum"=w1061:refnum<file>, "error out"=w1060:errorcluster)  [unwired: 1 in]
        n244 = Close File(refnum=w1061, error in=w1060) -> (error out=w1023:errorcluster)  [unwired: 1 out]
        n245 = VISA Write(VISA resource name=w1025, write buffer=";:PAGE:SCON:STAN OFF;:PAGE:CHAN:VSU2:DIS;" ("write buffer (\"\")"), error in (no error)=w1023) -> (VISA resource name out=w1021:refnum<visa-resource-name>, error out=w1022:errorcluster)  [unwired: 1 out]
      }
      frame "#" {
        n246 = VISA Write(VISA resource name=w1090, write buffer=":DISP ON" ("write buffer (\"\")"), error in (no error)=w1089) -> (VISA resource name out=w1088:refnum<visa-resource-name>, error out=w1087:errorcluster)  [unwired: 1 out]
      }
      frame "stressV" {
        n247 = Number To Decimal String(number=w1108) -> (decimal integer string=w1149:string)  [unwired: 1 in]
        n248 = Fract/Exp String To Number(string=w1146) -> (number=w1119:dbl[])  [unwired: 3 in, 1 out]
        n249 = Concatenate Strings(w1133, "-stressV-" ("Substring"), w1149, w1107, ".txt" ("Substring")) -> (w1147:string)
        n250 = String To Path(string=w1147) -> (path=w1137:path)
        n251 = Index Array(array=w1119, index=3 ("Index")) -> (element=w1116:dbl)
        n252 = Index Array(array=w1119, index=1 ("Index")) -> (element=w1114:dbl)
        n253 = Index Array(array=w1119, index=0 ("Index")) -> (element=w1113:dbl)
        n254 = Index Array(array=w1119, index=4 ("Index")) -> (element=w1118:dbl)
        n255 = Index Array(array=w1119, index=2 ("Index")) -> (element=w1115:dbl)
        n256 = call "4155C Config V Stress.vi"("VISA session"=w1152, "ID compliance"=w1116, "VD"=w1114, "VG"=w1113, "IG compliance"=w1115, "error in (no error)"=w1151, "Display on/off"=TRUE) -> ("dup VISA resource name"=w1154:refnum<visa-resource-name>, "error out"=w1153:errorcluster)
        n257 = call "4155C Apply Stress.vi"("error in (no error)"=w1153, "Duration"=w1118, "Emergency Stop"=w1132, "VISA resource name in"=w1154) -> ("error out"=w1130:errorcluster, "VISA Resource Name out"=w1128:refnum<visa-resource-name>)
        n258 = VISA Write(VISA resource name=w1128, write buffer=":DISP ON" ("write buffer (\"\")"), error in (no error)=w1130) -> (VISA resource name out=w1127:refnum<visa-resource-name>, error out=w1129:errorcluster)  [unwired: 1 out]
        n259 = call <vilib>:"compatOverwrite.vi"("overwrite (F)"=TRUE) -> ("overwrite?"=w1112:T7)
        n260 = Open/Create/Replace File(file path (use dialog)=w1137, error in=w1129, operation (0:open)=w1112) -> (refnum out=w1140:refnum<file>, error out=w1139:errorcluster)  [unwired: 3 in, 1 out]
        n261 = call "4155C Write array to file.vi"("Byte Stream File Refnum"=w1140, "Header"=string[] ["V stress completed successfully", ""], "error in (no error)"=w1139) -> ("dup refnum"=w1142:refnum<file>, "error out"=w1141:errorcluster)  [unwired: 2 in]
        n262 = Close File(refnum=w1142, error in=w1141) -> (error out=w1135:errorcluster)  [unwired: 1 out]
      }
      frame "stressI" {
        n263 = Number To Decimal String(number=w1164) -> (decimal integer string=w1201:string)  [unwired: 1 in]
        n264 = Fract/Exp String To Number(string=w1198) -> (number=w1173:dbl[])  [unwired: 3 in, 1 out]
        n265 = Concatenate Strings(w1185, "-stressI-" ("Substring"), w1201, w1163, ".txt" ("Substring")) -> (w1199:string)
        n266 = String To Path(string=w1199) -> (path=w1189:path)
        n267 = Index Array(array=w1173, index=1 ("Index")) -> (element=w1169:dbl)
        n268 = Index Array(array=w1173, index=0 ("Index")) -> (element=w1170:dbl)
        n269 = call "4155C Config I Stress.vi"("VISA session"=w1204, "IDG"=w1170, "VDG compliance"=w1169, "error in (no error)"=w1203, "Display on/off"=TRUE) -> ("dup VISA resource name"=w1206:refnum<visa-resource-name>, "error out"=w1205:errorcluster)
        n270 = Index Array(array=w1173, index=2 ("Index")) -> (element=w1171:dbl)
        n271 = call "4155C Apply Stress.vi"("error in (no error)"=w1205, "Duration"=w1171, "Emergency Stop"=w1184, "VISA resource name in"=w1206) -> ("error out"=w1182:errorcluster, "VISA Resource Name out"=w1180:refnum<visa-resource-name>)
        n272 = VISA Write(VISA resource name=w1180, write buffer=":DISP ON" ("write buffer (\"\")"), error in (no error)=w1182) -> (VISA resource name out=w1179:refnum<visa-resource-name>, error out=w1181:errorcluster)  [unwired: 1 out]
        n273 = call <vilib>:"compatOverwrite.vi"("overwrite (F)"=TRUE) -> ("overwrite?"=w1168:T7)
        n274 = Open/Create/Replace File(file path (use dialog)=w1189, error in=w1181, operation (0:open)=w1168) -> (refnum out=w1192:refnum<file>, error out=w1191:errorcluster)  [unwired: 3 in, 1 out]
        n275 = call "4155C Write array to file.vi"("Byte Stream File Refnum"=w1192, "Header"=string[] ["I stress completed successfully", ""], "error in (no error)"=w1191) -> ("dup refnum"=w1194:refnum<file>, "error out"=w1193:errorcluster)  [unwired: 2 in]
        n276 = Close File(refnum=w1194, error in=w1193) -> (error out=w1187:errorcluster)  [unwired: 1 out]
      }
      frame "vsu2pulse" {
        n277 = Number To Decimal String(number=w1216) -> (decimal integer string=w1251:string)  [unwired: 1 in]
        n278 = Fract/Exp String To Number(string=w1248) -> (number=w1224:dbl[])  [unwired: 3 in, 1 out]
        n279 = Concatenate Strings(w1236, "-vsu2-" ("Substring"), w1251, w1215, ".txt" ("Substring")) -> (w1249:string)
        n280 = String To Path(string=w1249) -> (path=w1240:path)
        n281 = Index Array(array=w1224, index=1 ("Index")) -> (element=w1223:dbl)
        n282 = Index Array(array=w1224, index=0 ("Index")) -> (element=w1221:dbl)
        n283 = call "4155C Config VSU2 Stress.vi"("error in (no error)"=w1253, "VSU2"=w1221, "Display on/off"=TRUE, "VISA session"=w1254) -> ("error out"=w1255:errorcluster, "dup VISA resource name"=w1256:refnum<visa-resource-name>)
        n284 = call "4155C Apply Stress.vi"("error in (no error)"=w1255, "Duration"=w1223, "Emergency Stop"=w1235, "VISA resource name in"=w1256) -> ("error out"=w1233:errorcluster, "VISA Resource Name out"=w1231:refnum<visa-resource-name>)
        n285 = VISA Write(VISA resource name=w1231, write buffer=":DISP ON" ("write buffer (\"\")"), error in (no error)=w1233) -> (VISA resource name out=w1230:refnum<visa-resource-name>, error out=w1232:errorcluster)  [unwired: 1 out]
        n286 = call <vilib>:"compatOverwrite.vi"("overwrite (F)"=TRUE) -> ("overwrite?"=w1220:T7)
        n287 = Open/Create/Replace File(file path (use dialog)=w1240, error in=w1232, operation (0:open)=w1220) -> (refnum out=w1243:refnum<file>, error out=w1242:errorcluster)  [unwired: 3 in, 1 out]
        n288 = call "4155C Write array to file.vi"("Byte Stream File Refnum"=w1243, "Header"=string[] ["VSU2 pulse completed successfully", ""], "error in (no error)"=w1242) -> ("dup refnum"=w1245:refnum<file>, "error out"=w1244:errorcluster)  [unwired: 2 in]
        n289 = Close File(refnum=w1245, error in=w1244) -> (error out=w1238:errorcluster)  [unwired: 1 out]
      }
      frame "sample-fpp" {
        w1277 = string[] ["Time /s", "Id VgVd /A", "Ig VgVd /A", "Vp1 VgVd /V", "Vp2 VgVd /V"] ("Header")
        w1281 = "%d" ("format string")
        n290 = Number To Decimal String(number=w1266) -> (decimal integer string=w1329:string)  [unwired: 1 in]
        n291 = Fract/Exp String To Number(string=w1326) -> (number=w1314:dbl[])  [unwired: 3 in, 1 out]
        n292 = Concatenate Strings(w1320, "-samplefpp-" ("Substring"), w1329, w1265, ".txt" ("Substring")) -> (w1327:string)
        n293 = String To Path(string=w1327) -> (path=w1289:path)
        n294 = Index Array(array=w1314, index=0 ("Index")) -> (element=w1275:dbl)
        n295 = Index Array(array=w1314, index=1 ("Index")) -> (element=w1274:dbl)
        n296 = Index Array(array=w1314, index=2 ("Index")) -> (element=w1322:dbl)
        n297 = Index Array(array=w1314, index=3 ("Index")) -> (element=w1312:dbl)
        n298 = call "4155C Config Sampling Measurements FPP.vi"("VISA session"=w1332, "Num Points"=w1322, "Vg"=w1275, "Display on/off"=TRUE, "Gate Compliance"=w1321, "Drain Compliance"=w1330, "Standby"="Standby", "error in (no error)"=w1331, "Timings"=w1319, "Vd"=w1274, "Sample time"=w1312) -> ("dup VISA resource name"=w1291:refnum<visa-resource-name>, "error out"=w1290:errorcluster)  [unwired: 3 in]
        n299 = Number To Decimal String(number=w1275) -> (decimal integer string=w1301:string)  [unwired: 1 in]
        n300 = call "4155C Take Sample FPP.vi"("VISA resource name in"=w1291, "error in (no error)"=w1290, "Emergency Stop"=w1292) -> ("Time"=w1296:dbl[], "Vp1"=w1306:dbl[], "VISA Resource Name out"=w1272:refnum<visa-resource-name>, "Ig"=w1294:dbl[], "Id"=w1295:dbl[], "Vp2"=w1304:dbl[], "error out"=w1293:errorcluster)  [unwired: 10 in]
        n301 = Insert Into Array(array=dbl[][] [] ("Input Array"), new element=w1296) -> (w1310:dbl[][])  [unwired: 2 in]
        n302 = Number To Decimal String(number=w1274) -> (decimal integer string=w1299:string)  [unwired: 1 in]
        n303 = Insert Into Array(array=w1310, new element=w1295) -> (w1309:dbl[][])  [unwired: 2 in]
        n304 = Concatenate Strings("(Vg = " ("Substring"), w1301, "V, Vd = " ("Substring"), w1299, "V)" ("Substring")) -> (w1297:string)
        n305 = Insert Into Array(array=w1309, new element=w1294) -> (w1308:dbl[][])  [unwired: 2 in]
        n306 = Insert Into Array(array=w1308, new element=w1306) -> (w1305:dbl[][])  [unwired: 2 in]
        n307 = Insert Into Array(array=w1305, new element=w1304) -> (w1273:dbl[][])  [unwired: 2 in]
        n308 = call <vilib>:"compatOverwrite.vi"("overwrite (F)"=TRUE) -> ("overwrite?"=w1270:T7)
        n309 = Open/Create/Replace File(file path (use dialog)=w1289, error in=w1293, operation (0:open)=w1270) -> (refnum out=w1286:refnum<file>, error out=w1287:errorcluster)  [unwired: 3 in, 1 out]
        n310 = Array To Spreadsheet String(array=w1277, 3:w1281) -> (spreadsheet string=w1283:string)  [unwired: 1 in]
        n311 = Transpose 2D Array(2D array=w1273) -> (transposed array=w1303:dbl[][])
        n312 = Search and Replace String(replace all?=TRUE ("replace all? (F)"), input string=w1283, search string="VgVd", replace string=w1297) -> (result string=w1279:string)  [unwired: 4 in, 3 out]
        n313 = Spreadsheet String To Array(format string=w1281, spreadsheet string=w1279, array type (2D Dbl)=w1277) -> (array=w1278:string[])  [unwired: 1 in]
        n314 = call "4155C Write array to file.vi"("Byte Stream File Refnum"=w1286, "Header"=w1278, "Data Array"=w1303, "error in (no error)"=w1287) -> ("dup refnum"=w1284:refnum<file>, "error out"=w1285:errorcluster)  [unwired: 1 in]
        n315 = Close File(refnum=w1284, error in=w1285) -> (error out=w1271:errorcluster)  [unwired: 1 out]
      }
      frame "resample-fpp" {
        w1355 = string[] ["Time /s", "Id VgVd /A", "Ig VgVd /A", "Vp1 VgVd /V", "Vp2 VgVd /V"] ("Header")
        w1359 = "%d" ("format string")
        n316 = Number To Decimal String(number=w1341) -> (decimal integer string=w1399:string)  [unwired: 1 in]
        n317 = Fract/Exp String To Number(string=w1396) -> (number=w1348:dbl[])  [unwired: 3 in, 1 out]
        n318 = Concatenate Strings(w1392, "-resamplefpp-" ("Substring"), w1399, w1342, ".txt" ("Substring")) -> (w1397:string)
        n319 = String To Path(string=w1397) -> (path=w1367:path)
        n320 = Index Array(array=w1348, index=0 ("Index")) -> (element=w1354:dbl)
        n321 = Index Array(array=w1348, index=1 ("Index")) -> (element=w1353:dbl)
        n322 = Number To Decimal String(number=w1354) -> (decimal integer string=w1377:string)  [unwired: 1 in]
        n323 = call "4155C Take Sample FPP.vi"("VISA resource name in"=w1350, "error in (no error)"=w1349, "Emergency Stop"=w1368) -> ("Time"=w1372:dbl[], "Vp1"=w1382:dbl[], "VISA Resource Name out"=w1352:refnum<visa-resource-name>, "Ig"=w1370:dbl[], "Id"=w1371:dbl[], "Vp2"=w1380:dbl[], "error out"=w1369:errorcluster)  [unwired: 10 in]
        n324 = Insert Into Array(array=dbl[][] [] ("Input Array"), new element=w1372) -> (w1386:dbl[][])  [unwired: 2 in]
        n325 = Number To Decimal String(number=w1353) -> (decimal integer string=w1375:string)  [unwired: 1 in]
        n326 = Insert Into Array(array=w1386, new element=w1371) -> (w1385:dbl[][])  [unwired: 2 in]
        n327 = Concatenate Strings("(Vg = " ("Substring"), w1377, "V, Vd = " ("Substring"), w1375, "V)" ("Substring")) -> (w1373:string)
        n328 = Insert Into Array(array=w1385, new element=w1370) -> (w1384:dbl[][])  [unwired: 2 in]
        n329 = Insert Into Array(array=w1384, new element=w1382) -> (w1381:dbl[][])  [unwired: 2 in]
        n330 = Insert Into Array(array=w1381, new element=w1380) -> (w1347:dbl[][])  [unwired: 2 in]
        n331 = call <vilib>:"compatOverwrite.vi"("overwrite (F)"=TRUE) -> ("overwrite?"=w1346:T7)
        n332 = Open/Create/Replace File(file path (use dialog)=w1367, error in=w1369, operation (0:open)=w1346) -> (refnum out=w1364:refnum<file>, error out=w1365:errorcluster)  [unwired: 3 in, 1 out]
        n333 = Array To Spreadsheet String(array=w1355, 3:w1359) -> (spreadsheet string=w1361:string)  [unwired: 1 in]
        n334 = Transpose 2D Array(2D array=w1347) -> (transposed array=w1379:dbl[][])
        n335 = Search and Replace String(replace all?=TRUE ("replace all? (F)"), input string=w1361, search string="VgVd", replace string=w1373) -> (result string=w1357:string)  [unwired: 4 in, 3 out]
        n336 = Spreadsheet String To Array(format string=w1359, spreadsheet string=w1357, array type (2D Dbl)=w1355) -> (array=w1356:string[])  [unwired: 1 in]
        n337 = call "4155C Write array to file.vi"("Byte Stream File Refnum"=w1364, "Header"=w1356, "Data Array"=w1379, "error in (no error)"=w1365) -> ("dup refnum"=w1362:refnum<file>, "error out"=w1363:errorcluster)  [unwired: 1 in]
        n338 = Close File(refnum=w1362, error in=w1363) -> (error out=w1351:errorcluster)  [unwired: 1 out]
      }
      frame "serial" {
        n339 = local read "Enable Termination\nChar (T)"() -> (w1417:bool)
        n340 = local read "Termination char\n(0xA = '\\n' = LF)\n(0xD = '\\r' = CR)"() -> (w1416:u8)
        n341 = Index Array(array=w1424, index=0 ("Index")) -> (element=w1423:string)
        n342 = local read "parity"() -> (w1407:u16)
        n343 = local read "Delay before read (ms)"() -> (w1418:u32)
        n344 = local read "byte count"() -> (w1415:u32)
        n345 = local read "Timeout (ms)"() -> (w1414:u32)
        n346 = local read "VISA resource name"() -> (w1411:refnum<visa-resource-name>)
        n347 = local read "baud rate"() -> (w1410:u32)
        n348 = local read "Serial End Mode for Reads"() -> (w1409:u16)
        n349 = local read "data bits"() -> (w1408:u16)
        n350 = local read "stop bits"() -> (w1413:u16)
        n351 = local read "flow control"() -> (w1412:u16)
        n352 = call "Serial write and read v0.5.vi"("Delay before read (ms)"=w1418, "Termination char\n(0xA = '\\n' = LF)\n(0xD = '\\r' = CR)"=w1416, "Enable Termination\nChar (T)"=w1417, "parity"=w1407, "stop bits"=w1413, "string to write"=w1423, "flow control"=w1412, "byte count"=w1415, "Serial Settings:Serial End Mode for Reads"=w1409, "Timeout (ms)"=w1414, "error in (no error)"=w1429, "VISA resource name"=w1411, "baud rate"=w1410, "data bits"=w1408) -> ("Serial port output"=w1419:string, "error out"=w1428:errorcluster)
        n353 = Build Array (concatenate)(w1419, w1420) -> (w1421:string[])
      }
      frame "pump" {
        # "Time array for valve position"
        # "Valve position"
        # "Time array for absolute plunger position"
        # "Absolute plunger position"
        # "Remove \"_\""
        # "Check if hard stop is pressed."
        # "Check if halt is pressed."
        # "Check if pump is idle. Else halt."
        n354 = local read "Hard stop pump"() -> (w1462:bool)
        n355 = local read "Halt pump"() -> (w1465:bool)
        n356 = local read "Enable Termination\nChar (T)"() -> (w1479:bool)
        n357 = local read "Termination char\n(0xA = '\\n' = LF)\n(0xD = '\\r' = CR)"() -> (w1478:u8)
        n358 = Index Array(array=w1483, index=0 ("Index")) -> (element=w1460:string)
        n359 = case shown="\"Initialization\"" w1458 {
          tunnel: w1460 -> [w1519 _ w1521 w1522 w1523 w1524 _ _ w1527 w1528 _]
          tunnel: [w1519 "/1H" w1521 w1522 w1523 w1524 "/1H" "/1H" w1527 w1528 "/1H"] -> w1459
          frame "No error", Default {
          }
          frame "Initialization" {
          }
          frame "Invalid command" {
          }
          frame "Invalid operand" {
          }
          frame "Device not initialized" {
          }
          frame "Internal failure" {
          }
          frame "Plunger overload" {
          }
          frame "Valve overload" {
          }
          frame "Plunger move not allowed" {
          }
          frame "A/D converter failure" {
          }
          frame "Command overflow" {
          }
        }
        n360 = case shown="True" w1465 {
          tunnel: [w1533 "/1H"] -> w1464
          tunnel: w1459 -> [w1533 _]
          frame False {
          }
          frame True {
            n361 = local write "Halt pump"(FALSE) -> ()
          }
        }
        n362 = case shown="True" w1462 {
          tunnel: [w1530 "/1T"] -> w1463
          tunnel: w1464 -> [w1530 _]
          frame False {
          }
          frame True {
            n363 = local write "Hard stop pump"(FALSE) -> ()
          }
        }
        n364 = local read "Serial End Mode for Reads"() -> (w1471:u16)
        n365 = local read "flow control"() -> (w1474:u16)
        n366 = local read "stop bits"() -> (w1475:u16)
        n367 = local read "parity"() -> (w1469:u16)
        n368 = local read "Delay before read (ms)"() -> (w1480:u32)
        n369 = local read "byte count"() -> (w1477:u32)
        n370 = local read "Timeout (ms)"() -> (w1476:u32)
        n371 = local read "VISA resource name"() -> (w1473:refnum<visa-resource-name>)
        n372 = local read "baud rate"() -> (w1472:u32)
        n373 = local read "data bits"() -> (w1470:u16)
        n374 = String Subset(string=w1454, offset (0)=1) -> (substring=w1452:string)  [unwired: 1 in]
        n375 = call "SPM Pump v0.6.vi"("Termination char\n(0xA = '\\n' = LF)\n(0xD = '\\r' = CR)"=w1478, "Enable Termination\nChar (T)"=w1479, "Timeout (ms)"=w1476, "Serial Settings:Serial End Mode for Reads"=w1471, "byte count"=w1477, "Delay before read (ms)"=w1480, "Time <input>"=w1457, "error in (no error)"=w1488, "Serial port input"=w1463, "VISA resource name"=w1473, "parity"=w1469, "baud rate"=w1472, "stop bits"=w1475, "data bits"=w1470, "flow control"=w1474, "Time units <input>"=w1452) -> ("Input command"=w1451:string, "Serial port data"=w1441:string[], "Pump status"=w1447:string, "Valve position"=w1449:i32, "Absolute plunger position"=w1461:i32, "Serial port"=w1456:string, "error out"=w1487:errorcluster)  [unwired: 1 in, 4 out]
        n376 = case shown="\"?\"" w1451 {
          tunnel: [w1500 w1508 w1514] -> w1468
          tunnel: w1467 -> [w1500 w1507 w1514]
          tunnel: w1461 -> [_ w1506 _]
          tunnel: w1448 -> [w1499 w1505 w1515]
          tunnel: [w1499 w1505 w1517] -> w1450
          tunnel: w1449 -> [_ _ w1516]
          tunnel: w1446 -> [_ w1504 w1512]
          tunnel: w1445 -> [w1498 w1503 w1513]
          tunnel: [w1498 w1502 w1513] -> w1444
          tunnel: [w1497 w1501 w1511] -> w1443
          tunnel: w1442 -> [w1497 w1501 w1510]
          frame "Q", Default {
          }
          frame "?" {
            n377 = Build Array (concatenate)(w1507, w1506) -> (w1508:i32[])
            n378 = Build Array (concatenate)(w1503, w1504) -> (w1502:i32[])
            n379 = call "4155C Split array.vi"("X data in"=w1502, "Y1 data in"=w1508) -> ("Array of clusters"=w1509:cluster{"Y data in":dbl[], "X data in":dbl[]}[])  [unwired: 5 in, 1 out]
            n380 = local write "Absolute plunger position vs time"(w1509) -> ()
          }
          frame "?6" {
            n381 = Build Array (concatenate)(w1515, w1516) -> (w1517:i32[])
            n382 = Build Array (concatenate)(w1510, w1512) -> (w1511:i32[])
            n383 = call "4155C Split array.vi"("X data in"=w1511, "Y1 data in"=w1517) -> ("Array of clusters"=w1518:cluster{"Y data in":dbl[], "X data in":dbl[]}[])  [unwired: 5 in, 1 out]
            n384 = local write "Valve position vs time"(w1518) -> ()
          }
        }
        n385 = Build Array (concatenate)(w1439, w1441) -> (w1440:string[][])
        n386 = Build Array (concatenate)(w1455, w1456) -> (w1481:string[])
      }
    }
    n387 = Build Array(w91, w136, w131) -> (w135:dbl[][])
    n388 = Build Array(w50, "Id max /A" ("VAR2 Name"), "Id min /A" ("VAR2 Name")) -> (w141:string[])
    n389 = Transpose 2D Array(2D array=w135) -> (transposed array=w134:dbl[][])
    n390 = Concatenate Strings(w69, "Prefix (Idmax-Idmin)", "Suffix (Idmax-Idmin)") -> (w148:string)
    n391 = Array To Spreadsheet String(array=w141, 3:"" ("format string")) -> (spreadsheet string=w140:string)  [unwired: 1 in]
    n392 = Array To Spreadsheet String(array=w134, 3:"%e" ("format string")) -> (spreadsheet string=w139:string)  [unwired: 1 in]
    n393 = String To Path(string=w148) -> (path=w147:path)
    n394 = Build Array(w140, w139) -> (w138:string[])
    n395 = Write to Text File(file (use dialog)=w147, text=w138, error in=w87) -> (refnum out=w149:refnum<file>, error out=w137:errorcluster)  [unwired: 1 in, 1 out]
    n396 = Close File(refnum=w149, error in=w137) -> (error out=w68:errorcluster)  [unwired: 1 out]
    n397 = Build Array(w64, w92) -> (w99:i32[][])
    n398 = Build Array(w50, "Absolute plunger position" ("VAR2 Name")) -> (w102:string[])
    n399 = Transpose 2D Array(2D array=w99) -> (transposed array=w90:i32[][])
    n400 = Array To Spreadsheet String(array=w102, 3:"" ("format string")) -> (spreadsheet string=w101:string)  [unwired: 1 in]
    n401 = Array To Spreadsheet String(array=w90, 3:"%e" ("format string")) -> (spreadsheet string=w98:string)  [unwired: 1 in]
    n402 = Build Array(w101, w98) -> (w104:string[])
    n403 = Concatenate Strings(w69, "Prefix (plunger)", "Suffix (plunger)") -> (w96:string)
    n404 = String To Path(string=w96) -> (path=w93:path)
    n405 = Write to Text File(file (use dialog)=w93, text=w104, error in=w68) -> (refnum out=w97:refnum<file>, error out=w106:errorcluster)  [unwired: 1 in, 1 out]
    n406 = Close File(refnum=w97, error in=w106) -> (error out=w67:errorcluster)  [unwired: 1 out]
    n407 = Concatenate Strings(w69, "Prefix (serial port log)", ".txt" ("Suffix")) -> (w114:string)
    n408 = String To Path(string=w114) -> (path=w111:path)
    n409 = Build Array(w50, "Serial port input" ("VAR2 Name"), "Pump status" ("VAR2 Name"), "Serial port output: ") -> (w54:string[])
    n410 = Array To Spreadsheet String(array=w60, 3:"" ("format string")) -> (spreadsheet string=w51:string)  [unwired: 1 in]
    n411 = Array To Spreadsheet String(array=w54, 3:"" ("format string")) -> (spreadsheet string=w52:string)  [unwired: 1 in]
    n412 = Build Array(w52, w51) -> (w53:string[])
    n413 = Array To Spreadsheet String(array=w59, 3:"" ("format string")) -> (spreadsheet string=w119:string)  [unwired: 1 in]
    n414 = Write to Text File(file (use dialog)=w111, text=w53, error in=w67) -> (refnum out=w115:refnum<file>, error out=w116:errorcluster)  [unwired: 1 in, 1 out]
    n415 = Close File(refnum=w115, error in=w116) -> (error out=w66:errorcluster)  [unwired: 1 out]
    n416 = local write "Serial port data"(w119) -> ()
    n417 = Build Array(w63, w71) -> (w79:i32[][])
    n418 = Build Array(w50, "Valve position" ("VAR2 Name")) -> (w82:string[])
    n419 = Transpose 2D Array(2D array=w79) -> (transposed array=w72:i32[][])
    n420 = Array To Spreadsheet String(array=w82, 3:"" ("format string")) -> (spreadsheet string=w81:string)  [unwired: 1 in]
    n421 = Array To Spreadsheet String(array=w72, 3:"%e" ("format string")) -> (spreadsheet string=w78:string)  [unwired: 1 in]
    n422 = Build Array(w81, w78) -> (w84:string[])
    n423 = Concatenate Strings(w69, "Prefix (valve)", "Suffix (valve)") -> (w76:string)
    n424 = String To Path(string=w76) -> (path=w73:path)
    n425 = Write to Text File(file (use dialog)=w73, text=w84, error in=w66) -> (refnum out=w77:refnum<file>, error out=w86:errorcluster)  [unwired: 1 in, 1 out]
    n426 = Close File(refnum=w77, error in=w86) -> (error out=w65:errorcluster)  [unwired: 1 out]
  }
  "error out" <- w9
